vi "CRYPost Processing.vi"(0 "Setup in":T1={"No.VI"=0, "Category"="", "StepName"="", "Seq setup flattened"="", "Comment"="", "Steps config."=[], "Jump config"=[], "Start"=0.0, "Increment"=0.0, "Name"="Pa", "Unit"="Pa", "Y data"=1, "Y prefix"="", "Y dB ref"=1.0, "Y unit"="", "Repeat State Array"=[]} {"Repeat State Array"."Start" format="%#_5g"; "Y dB ref" format="%.1f"; "Y data" items=["dB", "Lin"]; "Start" format="%#_5g"}, 5 "Data in":T4[](array[typedef]) {"Z data" items=["dB", "Lin"]; "X data" items=["dB", "Lin"]; "Y data" items=["dB", "Lin"]; "Z dB ref" format="%.1f"; "Z axis" items=["Log", "Lin"]; "X dB ref" format="%.1f"; "X axis" items=["Log", "Lin"]; "Y axis" items=["Log", "Lin"]; "Y dB ref" format="%.1f"; "Curve"."z" format="%.2f"; "Curve"."y" format="%.2f"; "Curve"."x" format="%.2f"}, 7 "Results in":T5 {"Margin" format="%.2f"}, 9 "Seq Setup in":string, 11 "Step name":string, 12 "Hardware in":string, 13 "Calibration in":string) -> (3 "Types Out":string[](array[string]), 4 "Inserted Names Out":string[](array[string]), 6 "Data out":T3 {"Z data" items=["dB", "Lin"]; "X data" items=["dB", "Lin"]; "Y data" items=["dB", "Lin"]; "Z dB ref" format="%.1f"; "Z axis" items=["Log", "Lin"]; "X dB ref" format="%.1f"; "X axis" items=["Log", "Lin"]; "Y axis" items=["Log", "Lin"]; "Y dB ref" format="%.1f"; "Curve"."z" format="%.2f"; "Curve"."y" format="%.2f"; "Curve"."x" format="%.2f"}, 8 "Result Out":T5 {"Margin" format="%.2f"}, 10 "Wave out":T7 {"Y dB ref" format="%.1f"; "Y axis" items=["Log", "Lin"]; "Y data" items=["dB", "Lin"]; "X data" items=["dB", "Lin"]})   [LabVIEW 2013]
uses:
  Typedef Control/CRYData Cluster.ctl
  Typedef Control/CRYResult Cluster Array.ctl
  Typedef Control/CRYResult Cluster.ctl
  Typedef Control/CRYWaveform Cluster Array.ctl
  Typedef Control/CRYWaveform Cluster.ctl
  Typedef Control/CRYData Cluster Array.ctl
  Typedef Control/CRYStep.ctl
  Task Sequence/CRYProject Run Control Global.vi
  CRYMainGlobal.vi
  SubVI/CRYPost Processing Global.vi
panel:
  in  "output cluster":T2
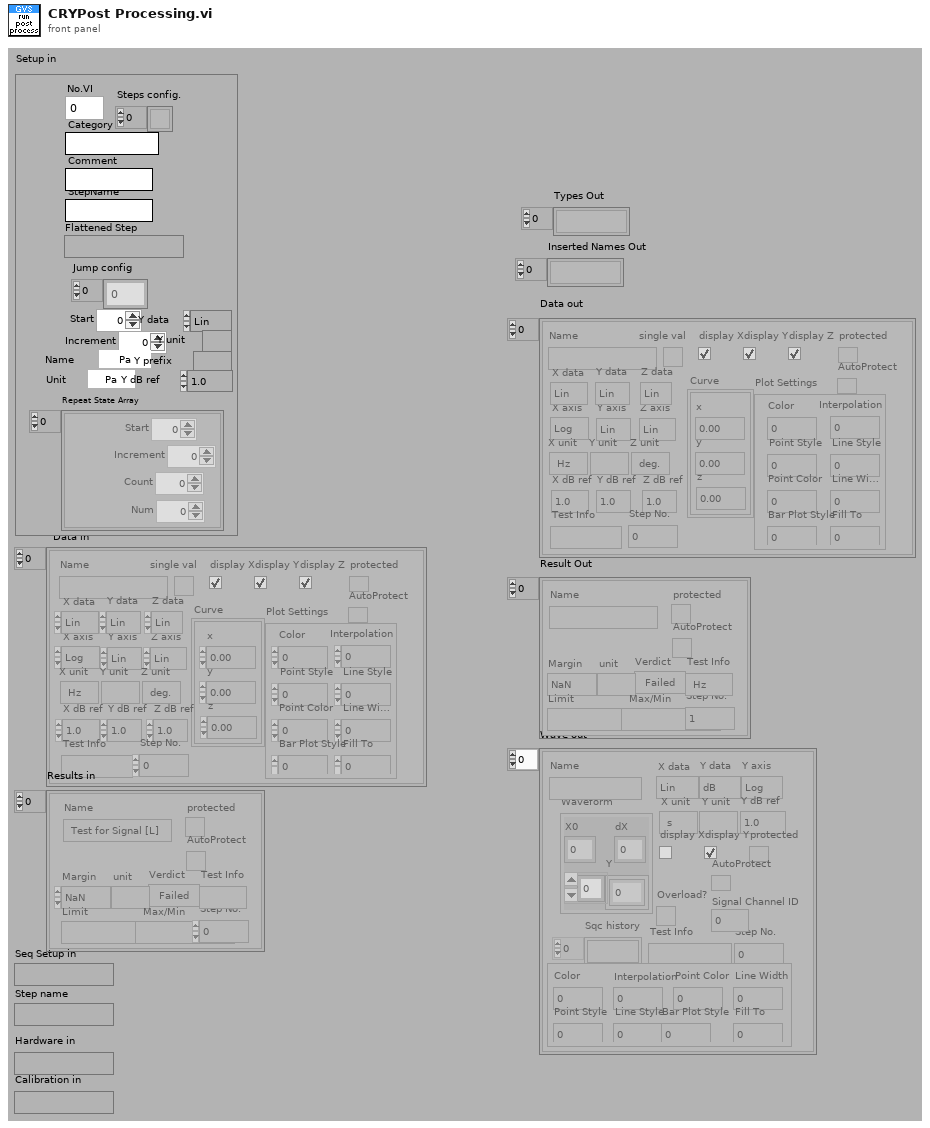
[diagram p1: front panel]
types:
  T1 = typedef "CRYStep.ctl" = cluster{"No.VI":i32, "Category":string, "StepName":string, "Seq setup flattened":string, "Comment":string, "Steps config.":bool[], "Jump config":i32[], "Start":dbl, "Increment":dbl, "Name":string, "Unit":string, "Y data":u16, "Y prefix":string, "Y dB ref":dbl, "Y unit":string, "Repeat State Array":cluster{"Start":dbl, "Increment":dbl, "Count":i32, "Num":i32}[]}
  T2 = cluster{"Res Name":string, "Type out":enum16{"Curves", "Values", "Results", "WFM"}}
  T3 = typedef "CRYData Cluster Array.ctl" = T4[]
  T4 = typedef "CRYData Cluster.ctl" = cluster{"Name":string, "Curve":cluster{"x":dbl, "y":dbl, "z":dbl}[], "X data":u16, "Y data":u16, "Z data":u16, "X axis":u16, "Y axis":u16, "Z axis":u16, "X unit":string, "Y unit":string, "Z unit":string, "X dB ref":dbl, "Y dB ref":dbl, "Z dB ref":dbl, "single val":bool, "protected":bool, "display X":bool, "display Y":bool, "display Z":bool, "Test Info":string, "Step No.":i32, "Plot Settings":cluster{"Color":u32, "Interpolation":u8, "Point Style":u8, "Line Style":u8, "Point Color":u32, "Line Width":u8, "Bar Plot Style":u8, "Fill To":i16}, "AutoProtect":bool}
  T5 = typedef "CRYResult Cluster Array.ctl" = T6[]
  T6 = typedef "CRYResult Cluster.ctl" = cluster{"Name":string, "Margin":dbl, "unit":string, "Verdict":bool, "Limit":string, "Max/Min":string, "protected":bool, "Step No.":i32, "Test Info":string, "AutoProtect":bool}
  T7 = typedef "CRYWaveform Cluster Array.ctl" = T8[]
  T8 = typedef "CRYWaveform Cluster.ctl" = cluster{"Waveform":cluster{"X0":dbl, "dX":dbl, "Y":sgl[]}, "X data":u16, "Y data":u16, "Y axis":u16, "X unit":string, "Y unit":string, "Y dB ref":dbl, "display Y":bool, "display X":bool, "Overload?":bool, "Test Info":string, "Step No.":i32, "Name":string, "protected":bool, "Sqc history":string[], "Signal Channel ID":i32, "Plot Settings":cluster{"Color":u32, "Interpolation":u8, "Point Style":u8, "Line Style":u8, "Point Color":u32, "Line Width":u8, "Bar Plot Style":u8, "Fill To":i16}, "AutoProtect":bool}
  T9 = cluster{"variant":variant, "Overwrite":bool, "Old Name":string, "New Name":string}
  T10 = cluster{"Start":dbl, "Increment":dbl, "Count":i32, "Num":i32}[]
  T11 = typedef "CRYPost Processing Cluster.ctl" = cluster{"Name":string, "Op Type":u16, "Curve A":string, "Curve B":string, "Axis Mode":u16, "Work Mode":u16, "Width":u16, "Weighting win":u16, "Search Mode":u16, "Freq Mode":u16, "New Sampling Rate":dbl, "Use Default Name":bool, "x":bool, "y":bool, "z":bool, "All points":bool, "A_single val axis":u16, "B_single val axis":u16, "Use Default Value":bool, "Result Name":string, "Smoothing Width":i32, "Window":u16, "Para_dB":sgl, "Para_%":sgl, "Exponent":sgl, "Hz":dbl, "Direct Weighting":bool, "Auto Inc":bool, "Inc(deg)":i32, "Total Rotation":i32, "Ref Freq Mode":u16, "Ref Waveform":string, "Sampling Rate":dbl, "Weighting Curve":string, "Ref Freq":dbl, "Curve Group":string[], "Search Items":string[], "Custom unit info":cluster{"use custom":bool, "lin/log":u16, "unit":string, "dB ref":dbl, "common dB":u16}, "Unit":string, "Type A":enum16{"Curves", "Values", "Results", "WFM"}, "Type B":enum16{"Curves", "Values", "Results", "WFM"}, "Unary Operator":u16, "Binary Operator":u16, "Statistical Operator":u16, "Constant ":dbl, "New Resolution":u16, "user equation cluster":T12, "Help":string, "Tab Value":enum32{"Setting", "Help"}, "Zwciker_X-axis":u16, "Zwicker_spectrum":bool, "Freq Sampling Mode":u16, "Freq Sampling Rate":dbl, "Smoothing":bool, "Work in Statics":u16, "Result Data":string[]}
  T12 = typedef "CRYUser Equation Cluster.ctl" = cluster{"Custom unit input array":cluster{"use custom":bool, "lin/log":u16, "unit":string, "dB ref":dbl, "common dB":u16}[], "Custom unit results array ":cluster{"use custom":bool, "lin/log":u16, "unit":string, "dB ref":dbl, "common dB":u16}[], "Desired Result Variables":string[], "Desired Result Names":string[], "Input Curve Names":string[], "Input Curve Variables":string[], "equation":string, "Input axis":u16[], "Results axis":u16[], "# input curves":i32, "# Desired result curves ":i32, "Input Values":string[], "Result Values":string[]}
  T13 = cluster{"Res Name":string, "Type out":enum16{"Curves", "Values", "Results", "WFM"}}[]
  T14 = enum16{"OK", "Yes", "YesNo", "YesNoCancel", "ReplaceAppend"}
  T15 = cluster{"variant":variant, "Overwrite":bool, "Old Name":string, "New Name":string}[]
  T16 = cluster{"use custom":bool, "lin/log":u16, "unit":string, "dB ref":dbl, "common dB":u16}
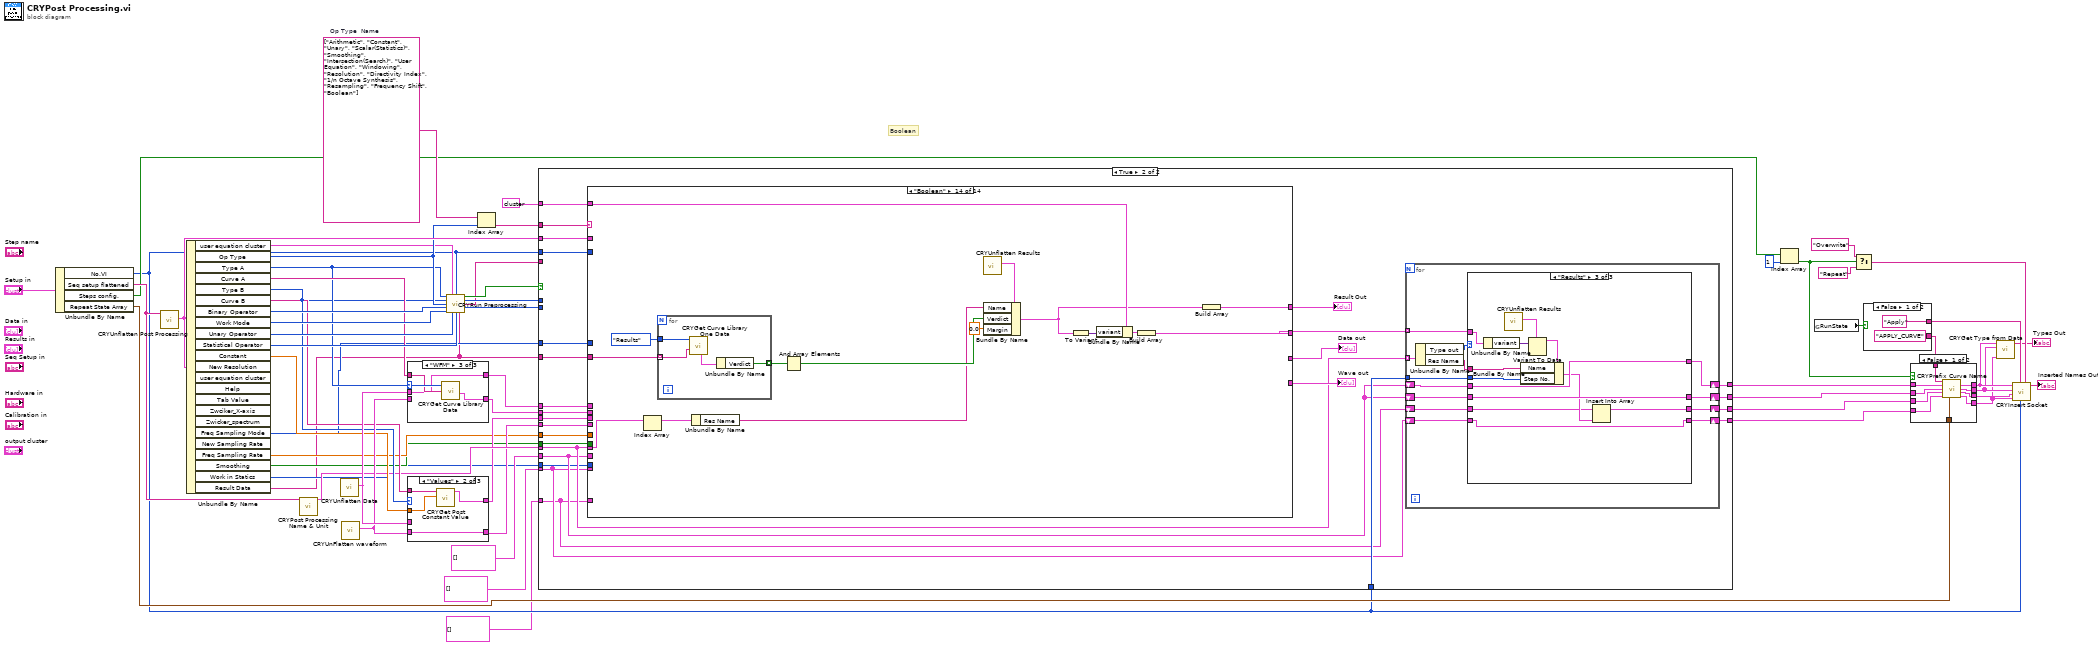
[diagram p0: block diagram]
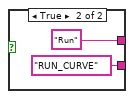
[diagram p2: hidden frame]
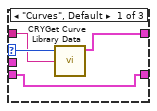
[diagram p4: hidden frame]
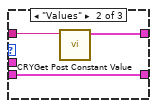
[diagram p5: hidden frame]
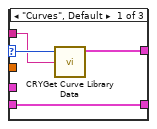
[diagram p6: hidden frame]
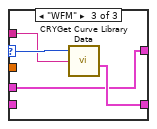
[diagram p7: hidden frame]
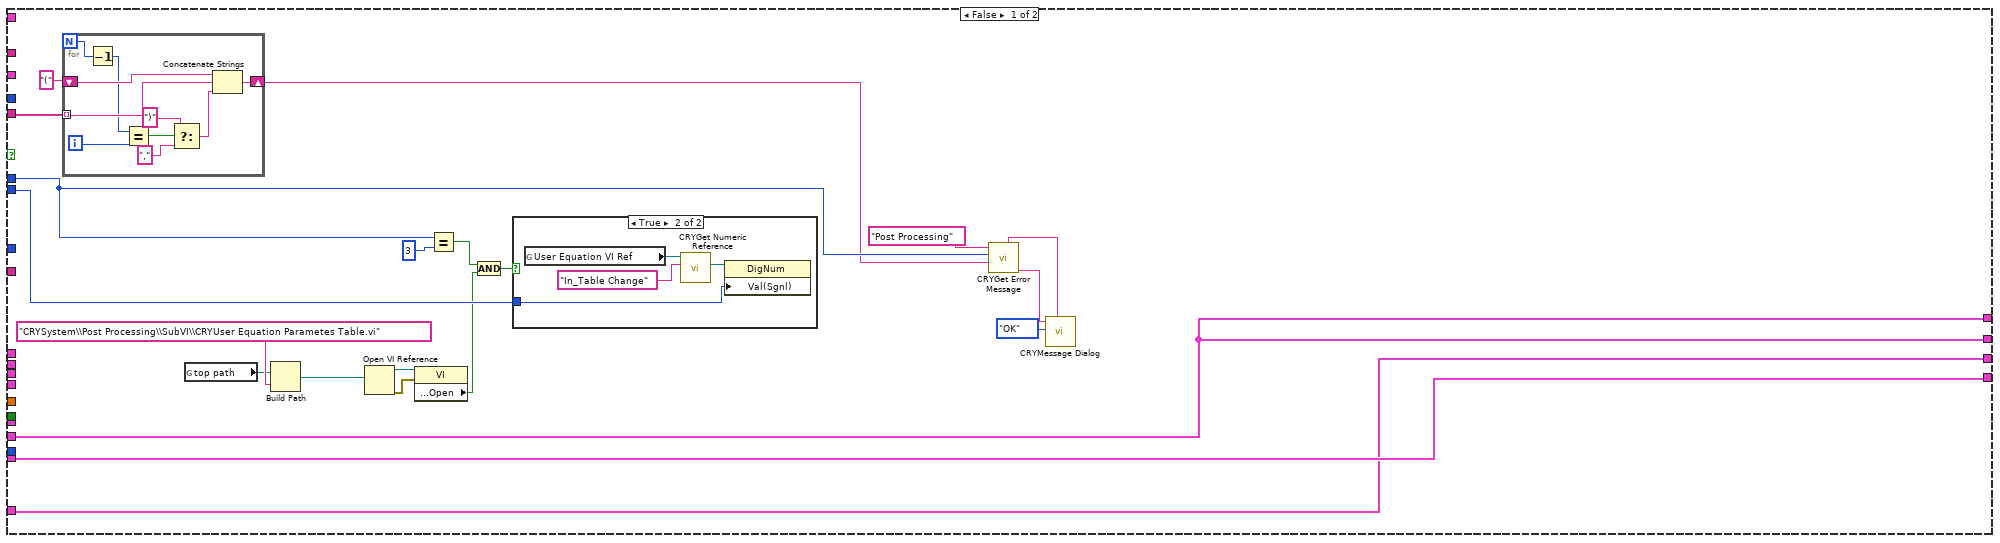
[diagram p8: hidden frame]
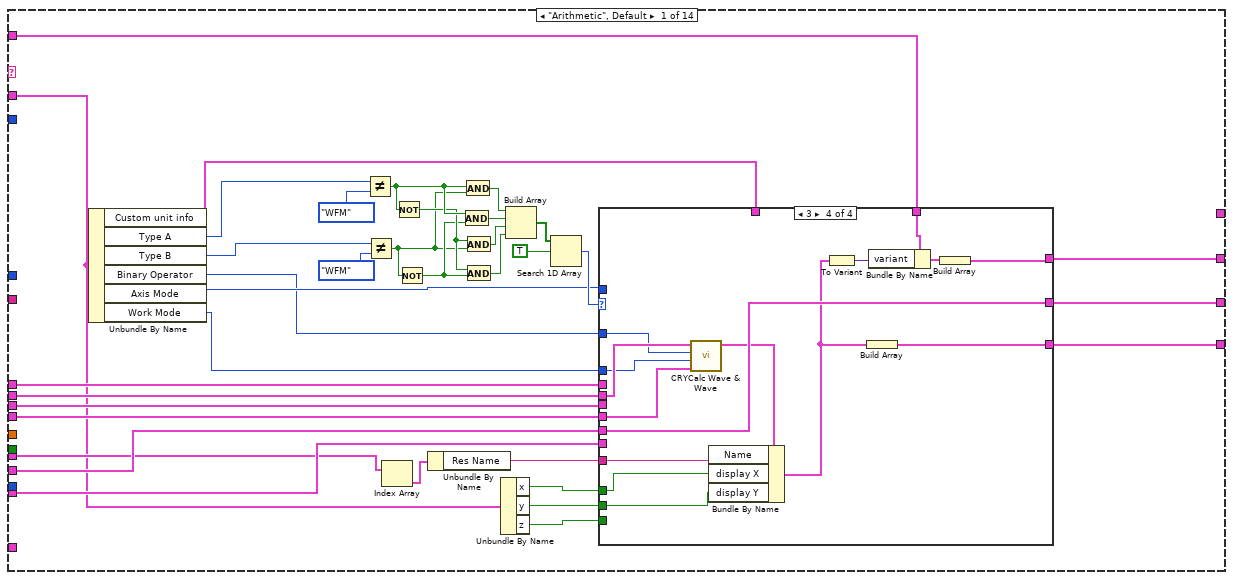
[diagram p10: hidden frame]
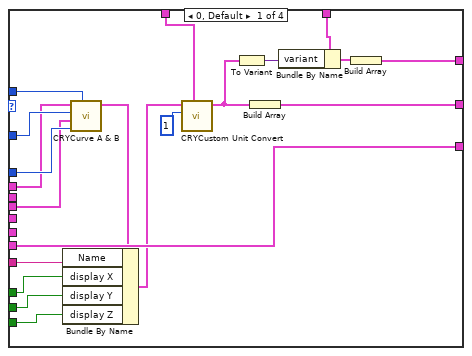
[diagram p11: hidden frame]
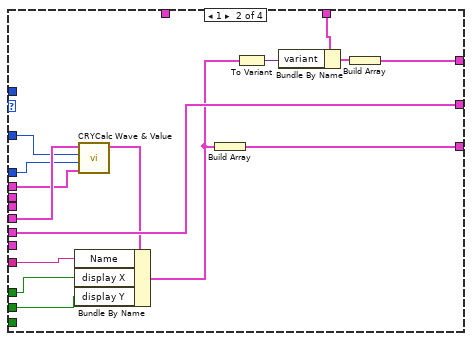
[diagram p12: hidden frame]
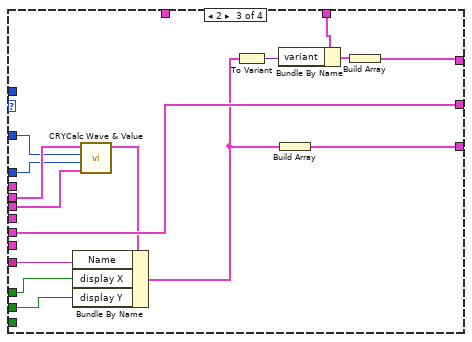
[diagram p13: hidden frame]
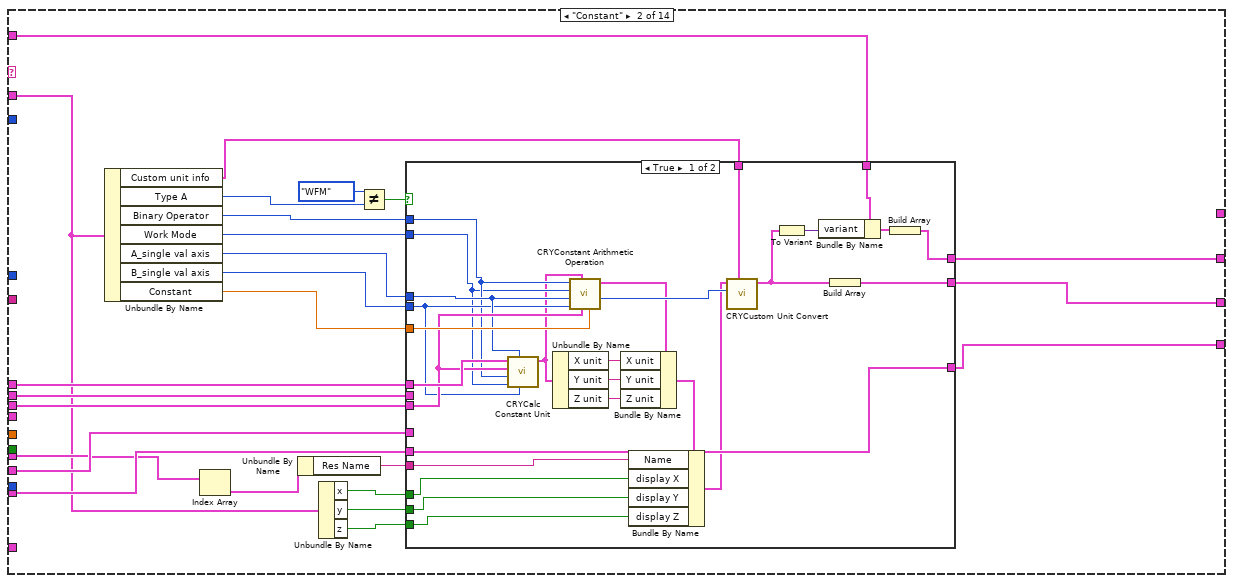
[diagram p14: hidden frame]
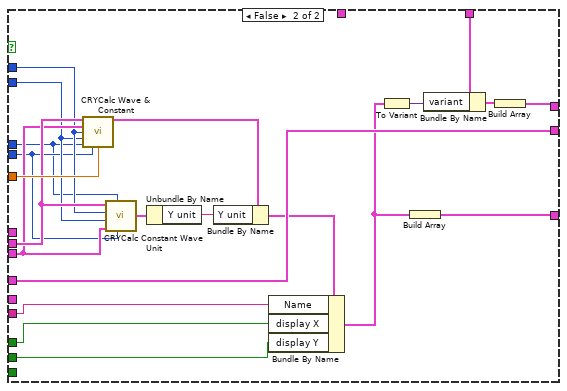
[diagram p15: hidden frame]
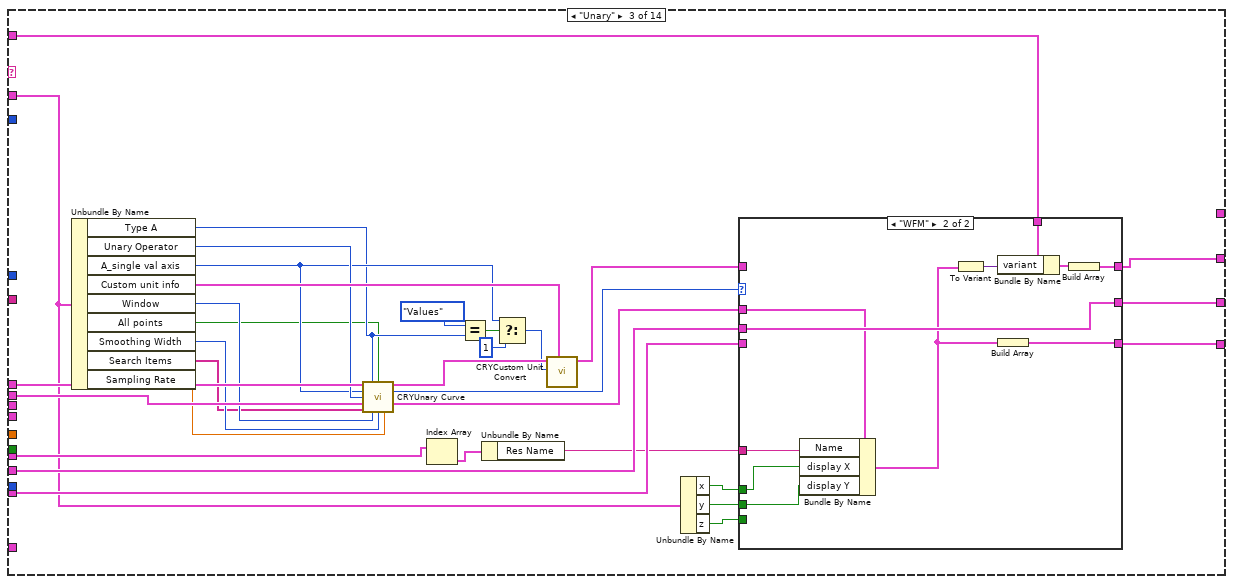
[diagram p16: hidden frame]
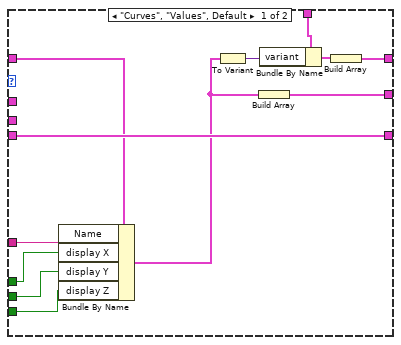
[diagram p17: hidden frame]
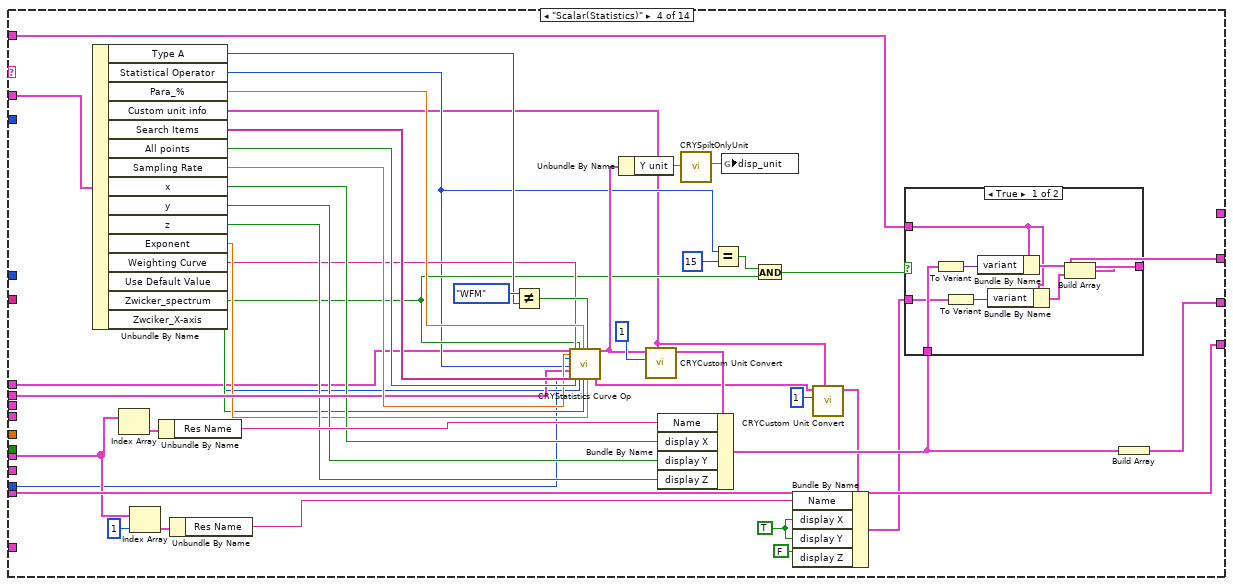
[diagram p18: hidden frame]
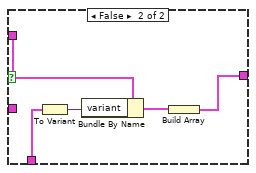
[diagram p19: hidden frame]
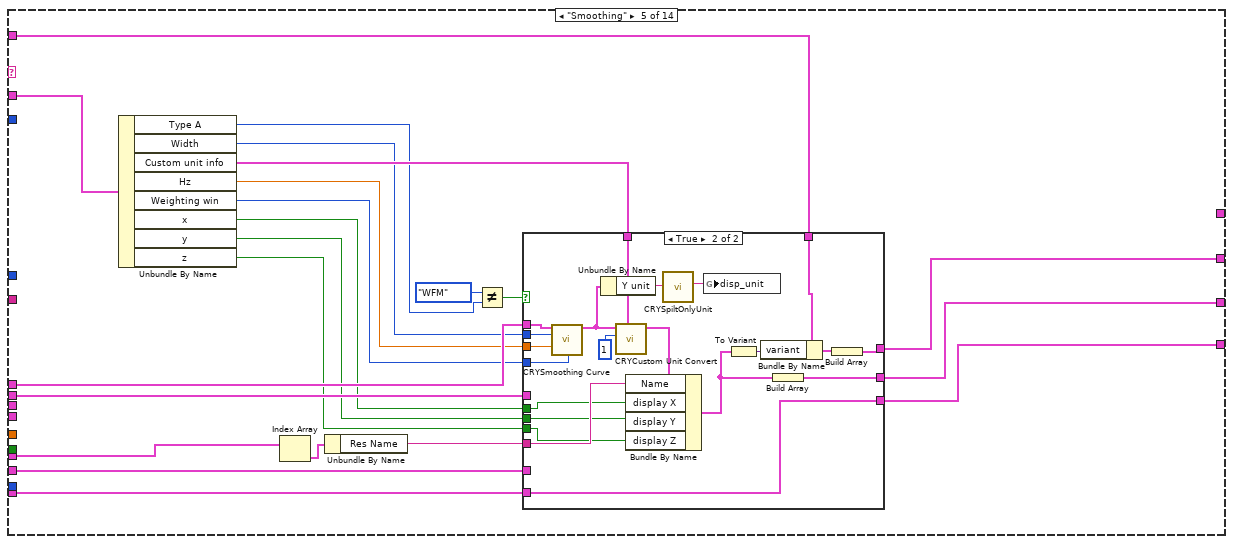
[diagram p20: hidden frame]
diagram:
  w56 = string[] ["Arithmetic", "Constant", "Unary", "Scalar(Statistics)", "Smoothing", "Intersection(Search)", "User Equation", "Windowing", "Resolution", "Directivity Index", "1/n Octave Synthesis", "Resampling", "Frequency Shift", "Boolean"]  # Op Type  Name
  # "Boolean"
  n1 = Unbundle By Name("Setup in") -> ("No.VI"=w9:i32, "Seq setup flattened"=w32:string, "Steps config."=w28:bool[], "Repeat State Array"=w18:T10)
  n2 = call "CRYUnflatten Post Processing.vi"("Unflatten Post Processing"=w32) -> ("Post-Processing"=w50:T11)  [unwired: 10 out]
  n3 = Unbundle By Name(w50) -> ("user equation cluster"=w47:T12, "Op Type"=w48:u16, "Type A"=w38:enum16{"Curves", "Values", "Results", "WFM"}, "Curve A"=w39:string, "Type B"=w36:enum16{"Curves", "Values", "Results", "WFM"}, "Curve B"=w37:string, "Binary Operator"=w55:u16, "Work Mode"=w54:u16, "Unary Operator"=w53:u16, "Statistical Operator"=w52:u16, "Constant"=w35:dbl, "Freq Sampling Mode"=w8:u16, "Freq Sampling Rate"=w7:dbl, "Smoothing"=w6:bool, "Work in Statics"=w5:u16, "Result Data"=w1:string[])  [unwired: 7 out]
  n4 = call "CRYPost Processing Name & Unit.vi"("Step setup"=w32) -> ("Result name and type"=w34:T13)  [unwired: 6 in, 4 out]
  n5 = call "CRYUnflatten Data.vi"() -> ("Datum"=w41:T4)  [unwired: 9 in, 2 out]
  n6 = call "CRYUnFlatten waveform.vi"() -> ("Waveform Cluster"=w40:T8)  [unwired: 9 in, 2 out]
  n7 = case shown="\"WFM\"" w38 {
    selector: w38 -> [w61 _ w68]
    tunnel: w39 -> [w60 w64 w67]
    tunnel: [w59 w63 w65] -> w26
    tunnel: w40 -> [w58 w62 _]
    tunnel: w41 -> [_ _ w65]
    tunnel: [w58 w62 w66] -> w25
    frame "Curves", Default {
      n8 = call "CRYGet Curve Library Data.vi"("Type"=w61, "Data Name"=w60) -> ("Curve"=w59:T4)  [unwired: 4 out]
    }
    frame "Values" {
      n9 = call "CRYGet Post Constant Value.vi"("Data Name"=w64) -> ("Value"=w63:T4)  [unwired: 2 in, 8 out]
    }
    frame "WFM" {
      n10 = call "CRYGet Curve Library Data.vi"("Type"=w68, "Data Name"=w67) -> ("Wave"=w66:T8)  [unwired: 4 out]
    }
  }
  n11 = case shown="\"Values\"" w36 {
    selector: w36 -> [w72 _ w80]
    tunnel: w37 -> [w71 w76 w79]
    tunnel: w35 -> [_ w75 _]
    tunnel: w41 -> [_ _ w77]
    tunnel: w40 -> [w69 w73 _]
    tunnel: [w70 w74 w77] -> w24
    tunnel: [w69 w73 w78] -> w23
    frame "Curves", Default {
      n12 = call "CRYGet Curve Library Data.vi"("Type"=w72, "Data Name"=w71) -> ("Curve"=w70:T4)  [unwired: 4 out]
    }
    frame "Values" {
      n13 = call "CRYGet Post Constant Value.vi"("Constant"=w75, "Data Name"=w76) -> ("Value"=w74:T4)  [unwired: 1 in, 8 out]
    }
    frame "WFM" {
      n14 = call "CRYGet Curve Library Data.vi"("Type"=w80, "Data Name"=w79) -> ("Wave"=w78:T8)  [unwired: 4 out]
    }
  }
  n15 = call "CRYRun Preprocessing.vi"("Type A"=w38, "user equation cluster"=w47, "No.VI"=w9, "Type B"=w36, "Type"=w48, "Binary Operator"=w55, "Work in"=w54, "Unary Operator"=w53, "Statistical Operator"=w52, "Result Data"=w1) -> ("Run Flag"=w51:bool, "Message Mode"=w49:u16, "Invalid Variable"=w46:string[], "index of Invalid"=w45:i32)  [unwired: 2 out]
  n16 = Index Array(array=w56, index=w48) -> (element=w57:string)
  n17 = case shown="True" w51 {
    tunnel: w57 -> [_ w141]
    tunnel: w50 -> [_ w140]
    tunnel: w26 -> [_ w139]
    tunnel: w25 -> [_ w138]
    tunnel: w24 -> [_ w137]
    tunnel: w23 -> [_ w136]
    tunnel: w49 -> [w96 _]
    tunnel: w46 -> [w100 _]
    tunnel: w45 -> [w98 _]
    tunnel: T4[] [] ("appended array") -> [w82 w126]
    tunnel: T8[] [] ("appended array") -> [w83 w125]
    tunnel: T9 {"variant"=variant, "Overwrite"=FALSE, "Old Name"="", "New Name"=""} ("Data") -> [_ w133]
    tunnel: w34 -> [_ w131]
    tunnel: [w82 w130] -> w22
    tunnel: [w82 w129] -> w21
    tunnel: [w83 w128] -> w20
    tunnel: w9 -> [_ w127]
    tunnel: w9 -> [_ w124]
    tunnel: w8 -> [_ w123]
    tunnel: w7 -> [_ w122]
    tunnel: w6 -> [_ w121]
    tunnel: w5 -> [_ w120]
    tunnel: T6[] [] ("appended array") -> [w81 w116]
    tunnel: [w81 w119] -> w3
    tunnel: w1 -> [_ w118]
    frame False {
      n18 = for {
        N -> [w112]
        tunnel: w100 -> [w115] mode=indexing
        shift-right: [w114] -> w92
        shift-left: "(" ("string") -> [w113]
        i -> [w111]
        n19 = Decrement(x=w112) -> (x-1=w110:i32)
        n20 = Equal?(x=w110, y=w111) -> (x = y?=w109:bool)
        n21 = Select(t=")", s=w109, f="," ("string")) -> (s? t:f=w106:string)
        n22 = Concatenate Strings(w113, w115, w106) -> (w114:string)
      }
      n23 = global read "CRYMainGlobal.vi" "top path"() -> (w89:path)
      n24 = Build Path(base path=w89, name or relative path="CRYSystem\\Post Processing\\SubVI\\CRYUser Equation Parametes Table.vi" ("StepName")) -> (appended path=w91:path)
      n25 = Open VI Reference(vi path=w91) -> (vi reference=w85:refnum<vi>, error out=w84:errorcluster)  [unwired: 1 in, 4 out]
      n26 = property class="VI"(reference=w85, error in=w84) -> ("Front Panel.Open"=w88:bool)  [unwired: 2 out]
      n27 = Equal?(x=w96, y=u16 3) -> (x = y?=w87:bool)
      n28 = And(x=w87, y=w88) -> (x .and. y?=w86:bool)
      n29 = case shown="True" w86 {
        tunnel: w98 -> [_ w102]
        frame False {
        }
        frame True {
          n30 = global read "CRYPost Processing Global.vi" "User Equation VI Ref"() -> (w105:refnum<vi>)
          n31 = call "CRYGet Numeric Reference.vi"("Label Name"="In_Table Change", "VI Refnum"=w105) -> ("Numeric Ref Out"=w103:refnum<vi>)  [unwired: 7 in, 2 out]
          n32 = property class="DigNum"(reference=w103, "Val(Sgnl)"=w102) -> ()  [unwired: 1 in, 2 out]
        }
      }
      n33 = call "CRYGet Error Message.vi"("String In"=w92, "Error No"=w96, "Kind"="Post Processing") -> ("Message Sub 3"=w95:string, "Window Title"=w94:string)  [unwired: 3 in, 4 out]
      n34 = call "CRYMessage Dialog.vi"("Window Title"=w94, "YesNoCancel"=T14."OK", "Message Content"=w95) -> ()  [unwired: 7 in, 2 out]
    }
    frame True {
      n35 = case shown="\"Boolean\"" w141 {
        tunnel: w140 -> [w145 w246 w318 w415 w450 w497 w563 w620 w751 w777 w799 w818 w873 _]
        tunnel: w139 -> [w159 w262 w343 w382 w449 w530 _ w617 w728 w755 w797 _ _ _]
        tunnel: w138 -> [w158 w261 w346 w408 w440 w511 _ w616 _ _ _ w811 w853 _]
        tunnel: w137 -> [w157 w260 _ _ _ w528 _ _ _ _ _ _ _ _]
        tunnel: w136 -> [w156 _ _ _ _ w512 _ _ _ _ _ _ _ _]
        tunnel: [w151 w256 w328 w404 w442 w508 w573 w611 w745 w774 w794 w817 w872 _] -> w135
        tunnel: [w155 w255 w326 w403 w439 w507 w567 w610 w744 w773 w793 w801 w850 _] -> w134
        tunnel: w126 -> [w152 w252 w325 _ w437 _ _ w613 _ _ _ w817 w868 _]
        tunnel: w125 -> [w153 w253 w327 w403 w438 w507 w567 w614 w744 w773 w793 w809 w867 _]
        tunnel: w133 -> [w150 w251 w330 w402 w436 w503 w572 w609 w741 w770 w790 w816 w871 w998]
        tunnel: [w149 w250 w329 w400 w435 w504 w571 w608 w740 w769 w789 w815 w870 w997] -> w132
        tunnel: w131 -> [w148 w249 w324 w377 w434 w502 _ w607 w739 w767 w787 w813 w857 w987]
        tunnel: w124 -> [_ _ _ _ _ _ w562 _ _ _ _ _ _ _]
        tunnel: w123 -> [_ _ _ _ _ _ _ _ _ _ _ _ w848 _]
        tunnel: w122 -> [_ _ _ _ _ _ _ _ _ _ _ _ w847 _]
        tunnel: w121 -> [_ _ _ _ _ _ _ _ w727 _ _ _ _ _]
        tunnel: w120 -> [_ _ _ w370 _ _ _ _ _ _ _ _ _ _]
        tunnel: w118 -> [_ _ _ _ _ _ _ _ _ _ _ _ _ w990]
        tunnel: [_ _ _ _ _ _ _ _ _ _ _ _ _ w992] -> w117
        tunnel: w116 -> [_ _ _ _ _ _ _ _ _ _ _ _ _ _]
        frame "Arithmetic", Default {
          n36 = Unbundle By Name(w145) -> ("Custom unit info"=w154:T16, "Type A"=w165:enum16{"Curves", "Values", "Results", "WFM"}, "Type B"=w164:enum16{"Curves", "Values", "Results", "WFM"}, "Binary Operator"=w161:u16, "Axis Mode"=w162:u16, "Work Mode"=w160:u16)
          n37 = Not Equal?(x=w165, y=enum16{"Curves", "Values", "Results", "WFM"}."WFM" ("Type A")) -> (x != y?=w174:bool)
          n38 = Not Equal?(x=w164, y=enum16{"Curves", "Values", "Results", "WFM"}."WFM" ("Type A")) -> (x != y?=w171:bool)
          n39 = Index Array(array=w148) -> (element=w147:T2)  [unwired: 1 in]
          n40 = Not(x=w174) -> (.not. x?=w173:bool)
          n41 = Not(x=w171) -> (.not. x?=w172:bool)
          n42 = Unbundle By Name(w147) -> ("Res Name"=w146:string)
          n43 = And(x=w174, y=w172) -> (x .and. y?=w170:bool)
          n44 = And(x=w174, y=w171) -> (x .and. y?=w177:bool)
          n45 = And(x=w173, y=w171) -> (x .and. y?=w169:bool)
          n46 = And(x=w173, y=w172) -> (x .and. y?=w168:bool)
          n47 = Unbundle By Name(w145) -> ("x"=w144:bool, "y"=w143:bool, "z"=w142:bool)
          n48 = Build Array(w177, w170, w169, w168) -> (w176:bool[])
          n49 = Search 1D Array(1D array=w176, element=TRUE) -> (index of element=w163:i32)  [unwired: 1 out]
          n50 = case shown="3" w163 {
            tunnel: w159 -> [w194 w211 _ _]
            tunnel: w158 -> [_ _ w227 w242]
            tunnel: w157 -> [w193 _ w226 _]
            tunnel: w156 -> [_ w212 _ w241]
            tunnel: w161 -> [w196 w210 w225 w240]
            tunnel: w162 -> [w197 _ _ _]
            tunnel: w160 -> [w195 w209 w224 w239]
            tunnel: w154 -> [w192 _ _ _]
            tunnel: [w189 w208 w223 w238] -> w155
            tunnel: [w190 w207 w222 w237] -> w151
            tunnel: w153 -> [w189 _ _ _]
            tunnel: w152 -> [_ w207 w222 w237]
            tunnel: w150 -> [w188 w204 w219 w234]
            tunnel: [w184 w203 w218 w233] -> w149
            tunnel: w146 -> [w182 w201 w216 w231]
            tunnel: w144 -> [w180 w199 w214 w229]
            tunnel: w143 -> [w179 w198 w213 w228]
            tunnel: w142 -> [w178 _ _ _]
            frame 0, Default {
              n51 = call "CRYCurve A & B.vi"("X-axis Combination"=w197, "Work in"=w195, "Curve B"=w193, "Operator"=w196, "Curve A"=w194) -> ("Result"=w183:T4)  [unwired: 6 out]
              n52 = Bundle By Name(cluster=w183, "Name"=w182, "display X"=w180, "display Y"=w179, "display Z"=w178) -> (w181:T4)
              n53 = call "CRYCustom Unit Convert.vi"("Custom unit info"=w192, "Axis Mode"=u16 1, "Data in"=w181) -> ("Data out"=w187:T4)  [unwired: 8 out]
              n54 = To Variant(anything=w187) -> (Variant=w186:variant)
              n55 = Build Array(w187) -> (w190:T4[])
              n56 = Bundle By Name(cluster=w188, "variant"=w186) -> (w185:T9)
              n57 = Build Array(w185) -> (w184:T15)
            }
            frame 1 {
              n58 = call "CRYCalc Wave & Value.vi"("Value in"=w211, "Work in"=w209, "Operator"=w210, "Wave in"=w212) -> ("Wave out"=w202:T8)  [unwired: 7 out]
              n59 = Bundle By Name(cluster=w202, "Name"=w201, "display X"=w199, "display Y"=w198) -> (w200:T8)
              n60 = Build Array(w200) -> (w208:T8[])
              n61 = To Variant(anything=w200) -> (Variant=w206:variant)
              n62 = Bundle By Name(cluster=w204, "variant"=w206) -> (w205:T9)
              n63 = Build Array(w205) -> (w203:T15)
            }
            frame 2 {
              n64 = call "CRYCalc Wave & Value.vi"("Value in"=w226, "Work in"=w224, "Operator"=w225, "Wave in"=w227) -> ("Wave out"=w217:T8)  [unwired: 7 out]
              n65 = Bundle By Name(cluster=w217, "Name"=w216, "display X"=w214, "display Y"=w213) -> (w215:T8)
              n66 = To Variant(anything=w215) -> (Variant=w221:variant)
              n67 = Bundle By Name(cluster=w219, "variant"=w221) -> (w220:T9)
              n68 = Build Array(w215) -> (w223:T8[])
              n69 = Build Array(w220) -> (w218:T15)
            }
            frame 3 {
              n70 = call "CRYCalc Wave & Wave.vi"("Wave in_2"=w241, "Work in"=w239, "Operator"=w240, "Wave in_1"=w242) -> ("Wave out"=w232:T8)  [unwired: 7 out]
              n71 = Bundle By Name(cluster=w232, "Name"=w231, "display X"=w229, "display Y"=w228) -> (w230:T8)
              n72 = To Variant(anything=w230) -> (Variant=w236:variant)
              n73 = Build Array(w230) -> (w238:T8[])
              n74 = Bundle By Name(cluster=w234, "variant"=w236) -> (w235:T9)
              n75 = Build Array(w235) -> (w233:T15)
            }
          }
        }
        frame "Constant" {
          n76 = Unbundle By Name(w246) -> ("Custom unit info"=w254:T16, "Type A"=w266:enum16{"Curves", "Values", "Results", "WFM"}, "Binary Operator"=w264:u16, "Work Mode"=w263:u16, "A_single val axis"=w258:u16, "B_single val axis"=w257:u16, "Constant"=w259:dbl)
          n77 = Index Array(array=w249) -> (element=w248:T2)  [unwired: 1 in]
          n78 = Unbundle By Name(w248) -> ("Res Name"=w247:string)
          n79 = Unbundle By Name(w246) -> ("x"=w245:bool, "y"=w244:bool, "z"=w243:bool)
          n80 = Not Equal?(x=enum16{"Curves", "Values", "Results", "WFM"}."WFM" ("Type A"), y=w266) -> (x != y?=w265:bool)
          n81 = case shown="True" w265 {
            tunnel: w262 -> [w291 _]
            tunnel: w261 -> [_ w303]
            tunnel: w260 -> [w290 w302]
            tunnel: w264 -> [w287 w301]
            tunnel: w263 -> [w286 w300]
            tunnel: w258 -> [w289 w298]
            tunnel: w257 -> [w288 w299]
            tunnel: w259 -> [w292 w314]
            tunnel: w254 -> [w293 _]
            tunnel: [w281 w312] -> w256
            tunnel: [w280 w313] -> w255
            tunnel: w253 -> [w280 _]
            tunnel: w252 -> [_ w312]
            tunnel: w251 -> [w277 w309]
            tunnel: [w275 w308] -> w250
            tunnel: w247 -> [w273 w307]
            tunnel: w245 -> [w271 w306]
            tunnel: w244 -> [w270 w305]
            tunnel: w243 -> [w269 _]
            frame True {
              n82 = call "CRYCalc Constant Unit.vi"("B_axis mode"=w288, "A_axis mode"=w289, "Work in"=w286, "Operator"=w287, "B data for units"=w290, "A data for units"=w291) -> ("Result out"=w268:T4)  [unwired: 5 in]
              n83 = Unbundle By Name(w268) -> ("X unit"=w284:string, "Y unit"=w283:string, "Z unit"=w282:string)
              n84 = call "CRYConstant Arithmetic Operation.vi"("Constant"=w292, "B data for units"=w290, "A data for units"=w268, "B_axis mode"=w288, "A_axis mode"=w289, "Work in"=w286, "Operator"=w287) -> ("Result out"=w285:T4)  [unwired: 4 in]
              n85 = Bundle By Name(cluster=w285, "X unit"=w284, "Y unit"=w283, "Z unit"=w282) -> (w274:T4)
              n86 = Bundle By Name(cluster=w274, "Name"=w273, "display X"=w271, "display Y"=w270, "display Z"=w269) -> (w272:T4)
              n87 = call "CRYCustom Unit Convert.vi"("Custom unit info"=w293, "Axis Mode"=w289, "Data in"=w272) -> ("Data out"=w276:T4)  [unwired: 8 out]
              n88 = To Variant(anything=w276) -> (Variant=w279:variant)
              n89 = Bundle By Name(cluster=w277, "variant"=w279) -> (w278:T9)
              n90 = Build Array(w276) -> (w281:T4[])
              n91 = Build Array(w278) -> (w275:T15)
            }
            frame False {
              n92 = call "CRYCalc Wave & Constant.vi"("Wave in"=w303, "Value in"=w302, "Operator"=w301, "Work in"=w300, "A_axis mode"=w298, "B_axis mode"=w299, "Constant"=w314) -> ("Wave out"=w296:T8)  [unwired: 8 out]
              n93 = call "CRYCalc Constant Wave Unit.vi"("B_axis mode"=w299, "A_axis mode"=w298, "Value in"=w302, "Work in"=w300, "Operator"=w301, "Wave in"=w303) -> ("Wave out"=w297:T8)  [unwired: 5 in]
              n94 = Unbundle By Name(w297) -> ("Y unit"=w295:string)
              n95 = Bundle By Name(cluster=w296, "Y unit"=w295) -> (w294:T8)
              n96 = Bundle By Name(cluster=w294, "Name"=w307, "display X"=w306, "display Y"=w305) -> (w304:T8)
              n97 = To Variant(anything=w304) -> (Variant=w311:variant)
              n98 = Build Array(w304) -> (w313:T8[])
              n99 = Bundle By Name(cluster=w309, "variant"=w311) -> (w310:T9)
              n100 = Build Array(w310) -> (w308:T15)
            }
          }
        }
        frame "Unary" {
          n101 = Unbundle By Name(w318) -> ("Type A"=w334:enum16{"Curves", "Values", "Results", "WFM"}, "Unary Operator"=w342:u16, "A_single val axis"=w337:u16, "Custom unit info"=w345:T16, "Window"=w341:u16, "All points"=w320:bool, "Smoothing Width"=w340:i32, "Search Items"=w321:string[], "Sampling Rate"=w319:dbl)
          n102 = call "CRYUnary Curve.vi"("Operand A"=w343, "Type A"=w334, "All points"=w320, "A _axis mode"=w337, "Unary Operator"=w342, "Wave in"=w346, "Search Items"=w321, "Win Mode"=w341, "Smoothing Width"=w340, "Sampling Rate"=w319) -> ("Result"=w344:T4, "Type out"=w333:enum16{"Curves", "Values", "Results", "WFM"}, "Wave out"=w331:T8)  [unwired: 3 out]
          n103 = Index Array(array=w324) -> (element=w323:T2)  [unwired: 1 in]
          n104 = Equal?(x=enum16{"Curves", "Values", "Results", "WFM"}."Values", y=w334) -> (x = y?=w338:bool)
          n105 = Unbundle By Name(w323) -> ("Res Name"=w322:string)
          n106 = Select(t=w337, s=w338, f=u16 1) -> (s? t:f=w335:u16)
          n107 = call "CRYCustom Unit Convert.vi"("Custom unit info"=w345, "Axis Mode"=w335, "Data in"=w344) -> ("Data out"=w332:T4)  [unwired: 8 out]
          n108 = Unbundle By Name(w318) -> ("x"=w317:bool, "y"=w316:bool, "z"=w315:bool)
          n109 = case shown="\"WFM\"" w333 {
            tunnel: w332 -> [w352 _]
            tunnel: w331 -> [_ w363]
            tunnel: w330 -> [w356 w367]
            tunnel: [w355 w366] -> w329
            tunnel: [w354 w364] -> w328
            tunnel: w327 -> [w353 _]
            tunnel: [w353 w365] -> w326
            tunnel: w325 -> [_ w364]
            tunnel: w322 -> [w351 w362]
            tunnel: w317 -> [w349 w360]
            tunnel: w316 -> [w348 w359]
            tunnel: w315 -> [w347 _]
            frame "Curves", "Values", Default {
              n110 = Bundle By Name(cluster=w352, "Name"=w351, "display X"=w349, "display Y"=w348, "display Z"=w347) -> (w350:T4)
              n111 = To Variant(anything=w350) -> (Variant=w358:variant)
              n112 = Build Array(w350) -> (w354:T4[])
              n113 = Bundle By Name(cluster=w356, "variant"=w358) -> (w357:T9)
              n114 = Build Array(w357) -> (w355:T15)
            }
            frame "WFM" {
              n115 = Bundle By Name(cluster=w363, "Name"=w362, "display X"=w360, "display Y"=w359) -> (w361:T8)
              n116 = To Variant(anything=w361) -> (Variant=w369:variant)
              n117 = Bundle By Name(cluster=w367, "variant"=w369) -> (w368:T9)
              n118 = Build Array(w361) -> (w365:T8[])
              n119 = Build Array(w368) -> (w366:T15)
            }
          }
        }
        frame "Scalar(Statistics)" {
          w374 = TRUE ("display Y")
          n120 = Unbundle By Name(w415) -> ("Type A"=w410:enum16{"Curves", "Values", "Results", "WFM"}, "Statistical Operator"=w386:u16, "Para_%"=w413:sgl, "Custom unit info"=w379:T16, "Search Items"=w414:string[], "All points"=w412:bool, "Sampling Rate"=w409:dbl, "x"=w397:bool, "y"=w396:bool, "z"=w395:bool, "Exponent"=w391:sgl, "Weighting Curve"=w390:string, "Use Default Value"=w389:bool, "Zwicker_spectrum"=w387:bool, "Zwciker_X-axis"=w388:u16)
          n121 = Index Array(array=w377) -> (element=w399:T2)  [unwired: 1 in]
          n122 = Index Array(array=w377, index=1) -> (element=w378:T2)
          n123 = Unbundle By Name(w399) -> ("Res Name"=w398:string)
          n124 = Unbundle By Name(w378) -> ("Res Name"=w375:string)
          n125 = Not Equal?(x=enum16{"Curves", "Values", "Results", "WFM"}."WFM" ("Type In"), y=w410) -> (x != y?=w407:bool)
          n126 = call "CRYStatistics Curve Op.vi"("Data in"=w382, "Sampling Rate"=w409, "work in statics"=w370, "Statistical Operator"=w386, "Wave"=w408, "Search range"=w414, "weight curve"=w390, "All points"=w412, "Zwicker_spectrum"=w387, "Zwicker_X-axis"=w388, "Para_Resonance(%)"=w413, "Use Default Value"=w389, "Curve/WFM ?"=w407, "Exponent"=w391) -> ("Ranged data out(Curve)"=w380:T4, "Ranged data out(Value)"=w393:T4)  [unwired: 8 in, 4 out]
          n127 = Unbundle By Name(w393) -> ("Y unit"=w392:string)
          n128 = call "CRYCustom Unit Convert.vi"("Custom unit info"=w379, "Axis Mode"=u16 1, "Data in"=w393) -> ("Data out"=w405:T4)  [unwired: 8 out]
          n129 = Bundle By Name(cluster=w405, "Name"=w398, "display X"=w397, "display Y"=w396, "display Z"=w395) -> (w401:T4)
          n130 = call "CRYSpiltOnlyUnit.vi"("In Unit String"=w392) -> ("Out Unit String"=w394:string)  [unwired: 10 in]
          n131 = Equal?(x=w386, y=u16 15) -> (x = y?=w384:bool)
          n132 = global write "CRYPost Processing Global.vi" "disp_unit"(w394) -> ()
          n133 = And(x=w384, y=w387) -> (x .and. y?=w383:bool)
          n134 = call "CRYCustom Unit Convert.vi"("Custom unit info"=w379, "Axis Mode"=u16 1, "Data in"=w380) -> ("Data out"=w373:T4)  [unwired: 8 out]
          n135 = Bundle By Name(cluster=w373, "Name"=w375, "display X"=w374, "display Y"=w374, "display Z"=FALSE) -> (w372:T4)
          n136 = case shown="True" w383 {
            tunnel: w402 -> [w416 w426]
            tunnel: w401 -> [w421 w425]
            tunnel: [w420 w424] -> w400
            tunnel: w372 -> [w418 _]
            frame True {
              n137 = To Variant(anything=w421) -> (Variant=w423:variant)
              n138 = To Variant(anything=w418) -> (Variant=w419:variant)
              n139 = Bundle By Name(cluster=w416, "variant"=w423) -> (w422:T9)
              n140 = Bundle By Name(cluster=w416, "variant"=w419) -> (w417:T9)
              n141 = Build Array(w422, w417) -> (w420:T15)
            }
            frame False {
              n142 = To Variant(anything=w425) -> (Variant=w428:variant)
              n143 = Bundle By Name(cluster=w426, "variant"=w428) -> (w427:T9)
              n144 = Build Array(w427) -> (w424:T15)
            }
          }
          n145 = Build Array(w401) -> (w404:T4[])
        }
        frame "Smoothing" {
          n146 = Unbundle By Name(w450) -> ("Type A"=w444:enum16{"Curves", "Values", "Results", "WFM"}, "Width"=w446:u16, "Custom unit info"=w448:T16, "Hz"=w447:dbl, "Weighting win"=w443:u16, "x"=w431:bool, "y"=w430:bool, "z"=w429:bool)
          n147 = Index Array(array=w434) -> (element=w433:T2)  [unwired: 1 in]
          n148 = Unbundle By Name(w433) -> ("Res Name"=w432:string)
          n149 = Not Equal?(x=enum16{"Curves", "Values", "Results", "WFM"}."WFM" ("Type In"), y=w444) -> (x != y?=w441:bool)
          n150 = case shown="True" w441 {
            tunnel: w449 -> [_ w487]
            tunnel: w448 -> [_ w486]
            tunnel: w447 -> [w464 w485]
            tunnel: w446 -> [_ w484]
            tunnel: w443 -> [w465 w483]
            tunnel: [w462 w481] -> w442
            tunnel: w440 -> [w466 _]
            tunnel: [w463 w480] -> w439
            tunnel: w438 -> [_ w480]
            tunnel: w437 -> [w462 _]
            tunnel: w436 -> [w459 w477]
            tunnel: [w458 w476] -> w435
            tunnel: w432 -> [w457 w474]
            tunnel: w431 -> [w455 w472]
            tunnel: w430 -> [w454 w471]
            tunnel: w429 -> [_ w470]
            frame False {
              n151 = call "CRYSmoothing Waveform.vi"("Weight Mode"=w465, "Width (s)"=w464, "Wave In"=w466) -> ("Wave out"=w451:T8)  [unwired: 8 in]
              n152 = Bundle By Name(cluster=w451, "display X"=w455, "display Y"=w454, "Name"=w457) -> (w456:T8)
              n153 = Unbundle By Name(w451) -> ("Y unit"=w452:string)
              n154 = call "CRYSpiltOnlyUnit.vi"("In Unit String"=w452) -> ("Out Unit String"=w453:string)  [unwired: 10 in]
              n155 = To Variant(anything=w456) -> (Variant=w461:variant)
              n156 = global write "CRYPost Processing Global.vi" "disp_unit"(w453) -> ()
              n157 = Bundle By Name(cluster=w459, "variant"=w461) -> (w460:T9)
              n158 = Build Array(w456) -> (w463:T8[])
              n159 = Build Array(w460) -> (w458:T15)
            }
            frame True {
              n160 = call "CRYSmoothing Curve.vi"("Data in"=w487, "Octav Mode"=w484, "Octave steps"=w485, "Weight Mode"=w483) -> ("Resulting data out"=w467:T4)  [unwired: 2 in, 9 out]
              n161 = Unbundle By Name(w467) -> ("Y unit"=w468:string)
              n162 = call "CRYCustom Unit Convert.vi"("Custom unit info"=w486, "Axis Mode"=u16 1, "Data in"=w467) -> ("Data out"=w475:T4)  [unwired: 8 out]
              n163 = Bundle By Name(cluster=w475, "Name"=w474, "display X"=w472, "display Y"=w471, "display Z"=w470) -> (w473:T4)
              n164 = call "CRYSpiltOnlyUnit.vi"("In Unit String"=w468) -> ("Out Unit String"=w469:string)  [unwired: 10 in]
              n165 = global write "CRYPost Processing Global.vi" "disp_unit"(w469) -> ()
              n166 = To Variant(anything=w473) -> (Variant=w478:variant)
              n167 = Bundle By Name(cluster=w477, "variant"=w478) -> (w479:T9)
              n168 = Build Array(w473) -> (w481:T4[])
              n169 = Build Array(w479) -> (w476:T15)
            }
          }
        }
        frame "Intersection(Search)" {
          n170 = Unbundle By Name(w497) -> ("Type A"=w517:enum16{"Curves", "Values", "Results", "WFM"}, "Type B"=w514:enum16{"Curves", "Values", "Results", "WFM"}, "Custom unit info"=w529:T16, "Search Items"=w493:string[], "All points"=w492:bool, "Search Mode"=w510:u16)
          n171 = Index Array(array=w502) -> (element=w501:T2)  [unwired: 1 in]
          n172 = Unbundle By Name(w501) -> ("Res Name"=w499:string)
          n173 = Not Equal?(x=w517, y=enum16{"Curves", "Values", "Results", "WFM"}."WFM" ("Type A")) -> (x != y?=w524:bool)
          n174 = Not Equal?(x=w514, y=enum16{"Curves", "Values", "Results", "WFM"}."WFM" ("Type A")) -> (x != y?=w521:bool)
          n175 = Not(x=w524) -> (.not. x?=w523:bool)
          n176 = Not(x=w521) -> (.not. x?=w522:bool)
          n177 = And(x=w524, y=w522) -> (x .and. y?=w520:bool)
          n178 = And(x=w524, y=w521) -> (x .and. y?=w527:bool)
          n179 = And(x=w523, y=w521) -> (x .and. y?=w519:bool)
          n180 = And(x=w523, y=w522) -> (x .and. y?=w518:bool)
          n181 = Build Array(w527, w520, w519, w518) -> (w526:bool[])
          n182 = Search 1D Array(1D array=w526, element=TRUE) -> (index of element=w513:i32)  [unwired: 1 out]
          n183 = case shown="1, 2" w513 {
            tunnel: w530 -> [w550 w555 _]
            tunnel: w528 -> [w551 _ _]
            tunnel: [w549 w554 w556] -> w491
            tunnel: w512 -> [_ _ w560]
            tunnel: w511 -> [_ _ w561]
            tunnel: w493 -> [w548 _ w558]
            tunnel: w492 -> [w547 _ w557]
            frame 0, Default {
              n184 = call "CRYSearch for Intersection.vi"("All points"=w547, "Search range"=w548, "Supress warnings (F)"=TRUE, "Operand B"=w551, "Operand A"=w550) -> ("Resulting data"=w549:T4)  [unwired: 6 out]
            }
            frame 1, 2 {
              n185 = Bundle By Name(cluster=w555, "Curve"=cluster{"x":dbl, "y":dbl, "z":dbl}[] [{"x"=nan, "y"=nan, "z"=nan}]) -> (w554:T4)
            }
            frame 3 {
              n186 = call "CRYSearch for Intersection of Wave.vi"("All points"=w557, "Search range"=w558, "Supress warnings (F)"=TRUE, "Waveform B"=w560, "Waveform A"=w561) -> ("Resulting data"=w556:T4)  [unwired: 6 in]
            }
          }
          n187 = case shown="0, Default" w510 {
            tunnel: w491 -> [w534 w541 w546]
            tunnel: [w532 w537 w544] -> w488
            frame 0, Default {
              n188 = Unbundle By Name(w534) -> ("Curve"=w536:cluster{"x":dbl, "y":dbl, "z":dbl}[])
              n189 = Index Array(array=w536) -> (element=w535:cluster{"x":dbl, "y":dbl, "z":dbl})  [unwired: 1 in]
              n190 = Build Array(w535) -> (w533:cluster{"x":dbl, "y":dbl, "z":dbl}[])
              n191 = Bundle By Name(cluster=w534, "single val"=TRUE, "Curve"=w533) -> (w532:T4)
            }
            frame 1 {
              n192 = Unbundle By Name(w541) -> ("Curve"=w543:cluster{"x":dbl, "y":dbl, "z":dbl}[])
              n193 = Reverse 1D Array(array=w543) -> (reversed array=w542:cluster{"x":dbl, "y":dbl, "z":dbl}[])
              n194 = Index Array(array=w542) -> (element=w540:cluster{"x":dbl, "y":dbl, "z":dbl})  [unwired: 1 in]
              n195 = Build Array(w540) -> (w539:cluster{"x":dbl, "y":dbl, "z":dbl}[])
              n196 = Bundle By Name(cluster=w541, "single val"=TRUE, "Curve"=w539) -> (w537:T4)
            }
            frame 2 {
              n197 = Bundle By Name(cluster=w546, "single val"=FALSE) -> (w544:T4)
            }
          }
          n198 = Unbundle By Name(w497) -> ("x"=w496:bool, "y"=w495:bool, "z"=w494:bool)
          n199 = Unbundle By Name(w488) -> ("Y unit"=w489:string)
          n200 = call "CRYCustom Unit Convert.vi"("Custom unit info"=w529, "Axis Mode"=u16 1, "Data in"=w488) -> ("Data out"=w500:T4)  [unwired: 8 out]
          n201 = Bundle By Name(cluster=w500, "Name"=w499, "display X"=w496, "display Y"=w495, "display Z"=w494) -> (w498:T4)
          n202 = call "CRYSpiltOnlyUnit.vi"("In Unit String"=w489) -> ("Out Unit String"=w490:string)  [unwired: 10 in]
          n203 = global write "CRYPost Processing Global.vi" "disp_unit"(w490) -> ()
          n204 = To Variant(anything=w498) -> (Variant=w506:variant)
          n205 = Bundle By Name(cluster=w503, "variant"=w506) -> (w505:T9)
          n206 = Build Array(w498) -> (w508:T4[])
          n207 = Build Array(w505) -> (w504:T15)
        }
        frame "User Equation" {
          n208 = global read "CRYMainGlobal.vi" "top path"() -> (w568:path)
          n209 = Build Path(base path=w568, name or relative path="CRYSystem\\Post Processing\\SubVI\\CRYUser Equation Parametes Table.vi" ("StepName")) -> (appended path=w570:path)
          n210 = Open VI Reference(vi path=w570) -> (vi reference=w565:refnum<vi>, error out=w564:errorcluster)  [unwired: 1 in, 4 out]
          n211 = property class="VI"(reference=w565, error in=w564) -> ("Front Panel.Open"=w566:bool)  [unwired: 2 out]
          n212 = stacked-sequence {
            tunnel: w563 -> [w586 _]
            tunnel: [w580 _] -> w573
            tunnel: w566 -> [w582 w597]
            tunnel: w563 -> [w579 _]
            tunnel: w562 -> [w578 _]
            frame #0 {
              n213 = Unbundle By Name(w586) -> ("user equation cluster"=w585:T12)
              n214 = call "CRYCalculate User Equation.vi"("No.VI"=w578, "User equation cluster In"=w585) -> ("Result Curves"=w581:T4[], "User equation cluster Out"=w584:T12)  [unwired: 7 in, 1 out]
              n215 = call "CRYFlatten User Equation Cluster.vi"("user equation cluster"=w584) -> ("Flatten String"=w583:string)  [unwired: 10 in]
              n216 = case shown="True" w582 {
                tunnel: w583 -> [_ w593]
                frame False {
                }
                frame True {
                  n217 = global read "CRYPost Processing Global.vi" "Post Editor VI Ref"() -> (w595:refnum<vi>)
                  n218 = call "CRYGet String Reference.vi"("Label Name"="User Equation String", "VI Refnum"=w595) -> ("String Ref Out"=w594:refnum<vi>)  [unwired: 9 out]
                  n219 = property class="Str"(reference=w594, "Val(Sgnl)"=w593) -> ()  [unwired: 1 in, 2 out]
                }
              }
              n220 = for {
                tunnel: w581 -> [w592] mode=indexing
                tunnel: [w591] -> w580 mode=indexing
                tunnel: w579 -> [w590]
                n221 = Unbundle By Name(w590) -> ("x"=w589:bool, "y"=w588:bool, "z"=w587:bool)
                n222 = Bundle By Name(cluster=w592, "display X"=w589, "display Y"=w588, "display Z"=w587) -> (w591:T4)
              }
            }
            frame #1 {
              n223 = case shown="True" w597 {
                frame False {
                }
                frame True {
                  n224 = global read "CRYPost Processing Global.vi" "User Equation VI Ref"() -> (w598:refnum<vi>)
                  n225 = call "CRYGet Boolean Reference.vi"("Label Name"=" Res_Table Change", "VI Refnum"=w598) -> ("Boolean Ref"=w600:refnum<vi>)  [unwired: 7 in, 2 out]
                  n226 = property class="Bool"(reference=w600, "Val(Sgnl)"=TRUE) -> ()  [unwired: 1 in, 2 out]
                }
              }
            }
          }
          n227 = for {
            tunnel: w573 -> [w576] mode=indexing
            tunnel: w572 -> [w575]
            tunnel: [w574] -> w571 mode=indexing
            n228 = To Variant(anything=w576) -> (Variant=w577:variant)
            n229 = Bundle By Name(cluster=w575, "variant"=w577) -> (w574:T9)
          }
        }
        frame "Windowing" {
          n230 = Unbundle By Name(w620) -> ("Custom unit info"=w615:T16, "Type A"=w612:enum16{"Curves", "Values", "Results", "WFM"}, "Search Items"=w618:string[], "All points"=w619:bool, "x"=w604:bool, "y"=w603:bool, "z"=w602:bool)
          n231 = Index Array(array=w607) -> (element=w606:T2)  [unwired: 1 in]
          n232 = Unbundle By Name(w606) -> ("Res Name"=w605:string)
          n233 = case shown="True" w619 {
            tunnel: w612 -> [w635 w692]
            tunnel: w617 -> [w634 w696]
            tunnel: w616 -> [w633 w695]
            tunnel: w618 -> [w632 _]
            tunnel: [w631 w694] -> w610
            tunnel: [w630 w693] -> w611
            tunnel: w615 -> [w629 w691]
            tunnel: w614 -> [w628 w690]
            tunnel: w613 -> [w627 w689]
            tunnel: w609 -> [w626 w688]
            tunnel: [w625 w687] -> w608
            tunnel: w605 -> [w624 w686]
            tunnel: w604 -> [w623 w685]
            tunnel: w603 -> [w622 w684]
            tunnel: w602 -> [w621 w683]
            frame False {
              n234 = case shown="\"Curves\", Default" w635 {
                tunnel: w634 -> [w655 _]
                tunnel: w633 -> [_ w675]
                tunnel: w632 -> [w658 w678]
                tunnel: [w649 w672] -> w631
                tunnel: [w650 w671] -> w630
                tunnel: w629 -> [w652 _]
                tunnel: w628 -> [w649 _]
                tunnel: w627 -> [_ w671]
                tunnel: w626 -> [w646 w668]
                tunnel: [w645 w667] -> w625
                tunnel: w624 -> [w643 w666]
                tunnel: w623 -> [w641 w664]
                tunnel: w622 -> [w640 w663]
                tunnel: w621 -> [w639 _]
                frame "Curves", Default {
                  n235 = Unbundle By Name(w655) -> ("Curve"=w659:cluster{"x":dbl, "y":dbl, "z":dbl}[], "X axis"=w657:u16)
                  n236 = Sort 1D Array(array=w659) -> (sorted array=w653:cluster{"x":dbl, "y":dbl, "z":dbl}[])
                  n237 = call "CRYCurve Cut to Range.vi"("Axis type (Lin)"=w657, "Range variable (x)"=enum16{"x", "y", "z"}."x", "Search range"=w658, "Curve in"=w653) -> ("Cut curve out"=w656:cluster{"x":dbl, "y":dbl, "z":dbl}[])  [unwired: 7 out]
                  n238 = Bundle By Name(cluster=w655, "Curve"=w656) -> (w636:T4)
                  n239 = call "CRYCustom Unit Convert.vi"("Custom unit info"=w652, "Axis Mode"=u16 1, "Data in"=w636) -> ("Data out"=w644:T4)  [unwired: 8 out]
                  n240 = Bundle By Name(cluster=w644, "Name"=w643, "display X"=w641, "display Y"=w640, "display Z"=w639) -> (w642:T4)
                  n241 = Unbundle By Name(w636) -> ("Y unit"=w637:string)
                  n242 = call "CRYSpiltOnlyUnit.vi"("In Unit String"=w637) -> ("Out Unit String"=w638:string)  [unwired: 10 in]
                  n243 = global write "CRYPost Processing Global.vi" "disp_unit"(w638) -> ()
                  n244 = To Variant(anything=w642) -> (Variant=w648:variant)
                  n245 = Bundle By Name(cluster=w646, "variant"=w648) -> (w647:T9)
                  n246 = Build Array(w642) -> (w650:T4[])
                  n247 = Build Array(w647) -> (w645:T15)
                }
                frame "WFM" {
                  n248 = call "CRYWaveform to DAT.vi"("Waveform In"=w675) -> ("Curve Out"=w676:T4)  [unwired: 10 out]
                  n249 = Unbundle By Name(w676) -> ("Curve"=w682:cluster{"x":dbl, "y":dbl, "z":dbl}[], "X axis"=w681:u16)
                  n250 = Sort 1D Array(array=w682) -> (sorted array=w673:cluster{"x":dbl, "y":dbl, "z":dbl}[])
                  n251 = Unbundle By Name(w675) -> ("Waveform.dX"=w674:dbl)
                  n252 = call "CRYCurve Cut to Range.vi"("Axis type (Lin)"=w681, "Range variable (x)"=enum16{"x", "y", "z"}."x", "Search range"=w678, "Curve in"=w673) -> ("Cut curve out"=w680:cluster{"x":dbl, "y":dbl, "z":dbl}[])  [unwired: 7 out]
                  n253 = Bundle By Name(cluster=w676, "Curve"=w680) -> (w677:T4)
                  n254 = call "CRYDAT to Waveform.vi"("dX"=w674, "Curve In"=w677) -> ("Waveform Out"=w660:T8)  [unwired: 9 out]
                  n255 = Bundle By Name(cluster=w660, "Name"=w666, "display X"=w664, "display Y"=w663) -> (w665:T8)
                  n256 = Unbundle By Name(w660) -> ("Y unit"=w661:string)
                  n257 = To Variant(anything=w665) -> (Variant=w670:variant)
                  n258 = call "CRYSpiltOnlyUnit.vi"("In Unit String"=w661) -> ("Out Unit String"=w662:string)  [unwired: 10 in]
                  n259 = Bundle By Name(cluster=w668, "variant"=w670) -> (w669:T9)
                  n260 = global write "CRYPost Processing Global.vi" "disp_unit"(w662) -> ()
                  n261 = Build Array(w665) -> (w672:T8[])
                  n262 = Build Array(w669) -> (w667:T15)
                }
              }
            }
            frame True {
              n263 = case shown="\"WFM\"" w692 {
                tunnel: w696 -> [w697 _]
                tunnel: w695 -> [_ w715]
                tunnel: [w710 w725] -> w694
                tunnel: [w711 w726] -> w693
                tunnel: w691 -> [w713 _]
                tunnel: w690 -> [w710 _]
                tunnel: w689 -> [_ w726]
                tunnel: w688 -> [w707 w722]
                tunnel: [w706 w721] -> w687
                tunnel: w686 -> [w704 w720]
                tunnel: w685 -> [w702 w719]
                tunnel: w684 -> [w701 w718]
                tunnel: w683 -> [w700 _]
                frame "Curves", Default {
                  n264 = call "CRYCustom Unit Convert.vi"("Custom unit info"=w713, "Axis Mode"=u16 1, "Data in"=w697) -> ("Data out"=w705:T4)  [unwired: 8 out]
                  n265 = Unbundle By Name(w697) -> ("Y unit"=w698:string)
                  n266 = Bundle By Name(cluster=w705, "Name"=w704, "display X"=w702, "display Y"=w701, "display Z"=w700) -> (w703:T4)
                  n267 = call "CRYSpiltOnlyUnit.vi"("In Unit String"=w698) -> ("Out Unit String"=w699:string)  [unwired: 10 in]
                  n268 = global write "CRYPost Processing Global.vi" "disp_unit"(w699) -> ()
                  n269 = To Variant(anything=w703) -> (Variant=w709:variant)
                  n270 = Bundle By Name(cluster=w707, "variant"=w709) -> (w708:T9)
                  n271 = Build Array(w703) -> (w711:T4[])
                  n272 = Build Array(w708) -> (w706:T15)
                }
                frame "WFM" {
                  n273 = Bundle By Name(cluster=w715, "Name"=w720, "display X"=w719, "display Y"=w718) -> (w714:T8)
                  n274 = Unbundle By Name(w714) -> ("Y unit"=w716:string)
                  n275 = To Variant(anything=w714) -> (Variant=w724:variant)
                  n276 = call "CRYSpiltOnlyUnit.vi"("In Unit String"=w716) -> ("Out Unit String"=w717:string)  [unwired: 10 in]
                  n277 = Build Array(w714) -> (w725:T8[])
                  n278 = Bundle By Name(cluster=w722, "variant"=w724) -> (w723:T9)
                  n279 = global write "CRYPost Processing Global.vi" "disp_unit"(w717) -> ()
                  n280 = Build Array(w723) -> (w721:T15)
                }
              }
            }
          }
        }
        frame "Resolution" {
          n281 = Unbundle By Name(w751) -> ("New Resolution"=w750:u16, "Freq Mode"=w749:u16, "Hz"=w748:dbl, "Custom unit info"=w746:T16, "x"=w734:bool, "y"=w733:bool, "z"=w732:bool)
          n282 = Index Array(array=w739) -> (element=w738:T2)  [unwired: 1 in]
          n283 = Unbundle By Name(w738) -> ("Res Name"=w736:string)
          n284 = call "CRYCurve Resolution.vi"("smoothing"=w727, "1/nOct_Hz"=w748, "Frequencies"=w749, "New Resolution"=w750, "Curve in"=w728) -> ("Curve out"=w729:T4)  [unwired: 6 out]
          n285 = call "CRYCustom Unit Convert.vi"("Custom unit info"=w746, "Axis Mode"=u16 1, "Data in"=w729) -> ("Data out"=w737:T4)  [unwired: 8 out]
          n286 = Unbundle By Name(w729) -> ("Y unit"=w730:string)
          n287 = Bundle By Name(cluster=w737, "Name"=w736, "display X"=w734, "display Y"=w733, "display Z"=w732) -> (w735:T4)
          n288 = call "CRYSpiltOnlyUnit.vi"("In Unit String"=w730) -> ("Out Unit String"=w731:string)  [unwired: 10 in]
          n289 = global write "CRYPost Processing Global.vi" "disp_unit"(w731) -> ()
          n290 = Build Array(w735) -> (w745:T4[])
          n291 = To Variant(anything=w735) -> (Variant=w743:variant)
          n292 = Bundle By Name(cluster=w741, "variant"=w743) -> (w742:T9)
          n293 = Build Array(w742) -> (w740:T15)
        }
        frame "Directivity Index" {
          n294 = Unbundle By Name(w777) -> ("Curve Group"=w754:string[], "Custom unit info"=w775:T16, "x"=w763:bool, "y"=w762:bool, "z"=w761:bool, "Weighting Curve"=w758:string, "Direct Weighting"=w759:bool, "Auto Inc"=w753:bool, "Inc(deg)"=w756:i32, "Total Rotation"=w752:i32)
          n295 = Index Array(array=w767) -> (element=w768:T2)  [unwired: 1 in]
          n296 = Unbundle By Name(w768) -> ("Res Name"=w765:string)
          n297 = call "CRYCalc Directivity Index.vi"("Weighting curve"=w758, "Direct_weight"=w759, "Inc(deg.)"=w756, "Total Rotation"=w752, "Curve Group"=w754, "Auto Inc"=w753, "Curve in"=w755) -> ("Curve out"=w757:T4)  [unwired: 4 out]
          n298 = call "CRYCustom Unit Convert.vi"("Custom unit info"=w775, "Axis Mode"=u16 1, "Data in"=w757) -> ("Data out"=w766:T4)  [unwired: 8 out]
          n299 = Bundle By Name(cluster=w766, "Name"=w765, "display X"=w763, "display Y"=w762, "display Z"=w761) -> (w764:T4)
          n300 = global write "CRYPost Processing Global.vi" "disp_unit"("") -> ()
          n301 = To Variant(anything=w764) -> (Variant=w772:variant)
          n302 = Build Array(w764) -> (w774:T4[])
          n303 = Bundle By Name(cluster=w770, "variant"=w772) -> (w771:T9)
          n304 = Build Array(w771) -> (w769:T15)
        }
        frame "1/n Octave Synthesis" {
          n305 = Unbundle By Name(w799) -> ("New Resolution"=w798:u16, "Custom unit info"=w796:T16, "x"=w783:bool, "y"=w782:bool, "z"=w781:bool)
          n306 = Index Array(array=w787) -> (element=w788:T2)  [unwired: 1 in]
          n307 = Unbundle By Name(w788) -> ("Res Name"=w785:string)
          n308 = call "CRYOctave synthesis.vi"("New Resolution"=w798, "Curve in"=w797) -> ("Curve out"=w778:T4)  [unwired: 1 in, 8 out]
          n309 = Unbundle By Name(w778) -> ("Y unit"=w779:string)
          n310 = call "CRYCustom Unit Convert.vi"("Custom unit info"=w796, "Axis Mode"=u16 1, "Data in"=w778) -> ("Data out"=w786:T4)  [unwired: 8 out]
          n311 = Bundle By Name(cluster=w786, "Name"=w785, "display X"=w783, "display Y"=w782, "display Z"=w781) -> (w784:T4)
          n312 = call "CRYSpiltOnlyUnit.vi"("In Unit String"=w779) -> ("Out Unit String"=w780:string)  [unwired: 10 in]
          n313 = global write "CRYPost Processing Global.vi" "disp_unit"(w780) -> ()
          n314 = Build Array(w784) -> (w794:T4[])
          n315 = To Variant(anything=w784) -> (Variant=w792:variant)
          n316 = Bundle By Name(cluster=w790, "variant"=w792) -> (w791:T9)
          n317 = Build Array(w791) -> (w789:T15)
        }
        frame "Resampling" {
          n318 = Unbundle By Name(w811) -> ("Name"=w810:string, "Waveform.Y"=w806:sgl[])
          n319 = Index Array(array=w813) -> (element=w814:T2)  [unwired: 1 in]
          n320 = Unbundle By Name(w814) -> ("Res Name"=w812:string)
          n321 = Empty String/Path?(string/path=w810) -> (empty?=w804:bool)
          n322 = Array Size(array=w806) -> (size(s)=w807:i32)
          n323 = Equal To 0?(x=w807) -> (x = 0?=w808:bool)
          n324 = Or(x=w804, y=w808) -> (x .or. y?=w805:bool)
          n325 = case shown="True" w805 {
            tunnel: w818 -> [w831 _]
            tunnel: [w830 w837] -> w801
            tunnel: w816 -> [w827 w834]
            tunnel: [w825 w836] -> w815
            tunnel: w812 -> [w824 w832]
            tunnel: w811 -> [w823 w833]
            tunnel: w809 -> [_ w837]
            tunnel: w804 -> [_ w835]
            frame False {
              n326 = Unbundle By Name(w831) -> ("y"=w822:bool, "x"=w821:bool, "New Sampling Rate"=w820:dbl)
              n327 = call "CRYWaveform Resampling.vi"("New Sampling Rate"=w820, "Wave"=w823) -> ("New Wave"=w819:T8)  [unwired: 9 in]
              n328 = Bundle By Name(cluster=w819, "display Y"=w822, "display X"=w821, "Name"=w824) -> (w826:T8)
              n329 = To Variant(anything=w826) -> (Variant=w829:variant)
              n330 = Bundle By Name(cluster=w827, "variant"=w829) -> (w828:T9)
              n331 = Build Array(w826) -> (w830:T8[])
              n332 = Build Array(w828) -> (w825:T15)
            }
            frame True {
              n333 = case shown="False" w835 {
                tunnel: [w842 T15 []] -> w836
                tunnel: w834 -> [w843 _]
                tunnel: w833 -> [w841 _]
                tunnel: w832 -> [w840 _]
                frame False {
                  w838 = TRUE ("display Y")
                  n334 = Bundle By Name(cluster=w841, "display Y"=w838, "display X"=w838, "Name"=w840) -> (w839:T8)
                  n335 = To Variant(anything=w839) -> (Variant=w845:variant)
                  n336 = Bundle By Name(cluster=w843, "variant"=w845) -> (w844:T9)
                  n337 = Build Array(w844) -> (w842:T15)
                }
                frame True {
                }
              }
            }
          }
          n338 = Index Array(array=w801) -> (element=w800:T8)  [unwired: 1 in]
          n339 = Unbundle By Name(w800) -> ("Y unit"=w802:string)
          n340 = call "CRYSpiltOnlyUnit.vi"("In Unit String"=w802) -> ("Out Unit String"=w803:string)  [unwired: 10 in]
          n341 = global write "CRYPost Processing Global.vi" "disp_unit"(w803) -> ()
        }
        frame "Frequency Shift" {
          # "++result=Playback sampling rate(Single Value)=zhunque ?"
          n342 = Unbundle By Name(w853) -> ("Name"=w869:string, "Waveform.Y"=w866:sgl[])
          n343 = Index Array(array=w857, index #1=0 ("index"), index #2=1 ("index")) -> (element #1=w858:T2, element #2=w861:T2)
          n344 = Empty String/Path?(string/path=w869) -> (empty?=w862:bool)
          n345 = Array Size(array=w866) -> (size(s)=w865:i32)
          n346 = Unbundle By Name(w861) -> ("Res Name"=w855:string)
          n347 = Unbundle By Name(w858) -> ("Res Name"=w856:string)
          n348 = Equal To 0?(x=w865) -> (x = 0?=w864:bool)
          n349 = Or(x=w862, y=w864) -> (x .or. y?=w863:bool)
          n350 = call "CRYUnflatten Data.vi"() -> ("Datum"=w854:T4)  [unwired: 9 in, 2 out]
          n351 = case shown="False" w863 {
            tunnel: w873 -> [w885 _]
            tunnel: [w884 w958] -> w872
            tunnel: [w883 w957] -> w850
            tunnel: w871 -> [w882 w952]
            tunnel: [w881 w962] -> w870
            tunnel: w868 -> [_ w960]
            tunnel: w867 -> [_ w959]
            tunnel: w862 -> [_ w961]
            tunnel: w856 -> [w880 w955]
            tunnel: w855 -> [w879 w954]
            tunnel: w854 -> [w878 w953]
            tunnel: w853 -> [w877 w956]
            tunnel: w848 -> [w874 _]
            tunnel: w847 -> [w875 _]
            frame False {
              n352 = Equal To 0?(x=w874) -> (x = 0?=w876:bool)
              n353 = case shown="True" w876 {
                tunnel: w885 -> [w889 w949]
                tunnel: [w894 w942] -> w884
                tunnel: [w893 w941] -> w883
                tunnel: w882 -> [w896 w937]
                tunnel: [w895 w935] -> w881
                tunnel: w880 -> [w892 w928]
                tunnel: w879 -> [w891 w927]
                tunnel: w878 -> [w897 w926]
                tunnel: w877 -> [w890 w925]
                tunnel: w875 -> [w888 w921]
                tunnel: w874 -> [w887 w920]
                frame False {
                  w902 = TRUE ("display Y")
                  w901 = FALSE ("display Y")
                  n354 = Unbundle By Name(w889) -> ("Ref Freq Mode"=w911:u16, "Ref Waveform"=w910:string, "Ref Freq"=w912:dbl)
                  n355 = case shown="0, Default" w911 {
                    tunnel: w910 -> [w917 _]
                    tunnel: [w917 ""] -> w899
                    frame 0, Default {
                    }
                    frame 1 {
                    }
                  }
                  n356 = call "CRYFrequency Shift.vi"("User Sampling Rate"=w888, "Freq Sampling Mode"=w887, "Reference Frequency"=w912, "Source Wave Name"=w899, "Waveform In"=w890) -> ("PlaybackSamplingRate"=w886:dbl, "Wave Out"=w904:T8)  [unwired: 5 in]
                  n357 = Bundle By Name(cluster=cluster{"x":dbl, "y":dbl, "z":dbl} {"x"=0.0, "y"=0.0, "z"=0.0}, "x"=w886) -> (w915:cluster{"x":dbl, "y":dbl, "z":dbl})
                  n358 = Build Array(w915) -> (w914:cluster{"x":dbl, "y":dbl, "z":dbl}[])
                  n359 = Bundle By Name(cluster=w897, "Curve"=w914, "single val"=TRUE, "Name"=w892, "display X"=TRUE, "display Y"=w901, "display Z"=w901, "X unit"="Hz") -> (w905:T4)
                  n360 = Bundle By Name(cluster=w904, "Name"=w891, "display X"=w902, "display Y"=w902) -> (w898:T8)
                  n361 = To Variant(anything=w905) -> (Variant=w908:variant)
                  n362 = To Variant(anything=w898) -> (Variant=w909:variant)
                  n363 = Bundle By Name(cluster=w896, "variant"=w908) -> (w907:T9)
                  n364 = Bundle By Name(cluster=w896, "variant"=w909) -> (w906:T9)
                  n365 = Build Array(w907, w906) -> (w895:T15)
                  n366 = Build Array(w905) -> (w894:T4[])
                  n367 = Build Array(w898) -> (w893:T8[])
                }
                frame True {
                  w931 = TRUE ("display Y")
                  w930 = FALSE ("display Y")
                  n368 = Unbundle By Name(w949) -> ("Ref Freq Mode"=w919:u16, "Ref Waveform"=w943:string, "Ref Freq"=w944:dbl)
                  n369 = case shown="1" w919 {
                    tunnel: w943 -> [w950 _]
                    tunnel: [w950 ""] -> w924
                    frame 0, Default {
                    }
                    frame 1 {
                    }
                  }
                  n370 = call "CRYFrequency Shift.vi"("User Sampling Rate"=w921, "Freq Sampling Mode"=w920, "Reference Frequency"=w944, "Source Wave Name"=w924, "Waveform In"=w925) -> ("PlaybackSamplingRate"=w923:dbl, "Wave Out"=w933:T8)  [unwired: 5 in]
                  n371 = Bundle By Name(cluster=cluster{"x":dbl, "y":dbl, "z":dbl} {"x"=0.0, "y"=0.0, "z"=0.0}, "x"=w923) -> (w947:cluster{"x":dbl, "y":dbl, "z":dbl})
                  n372 = Build Array(w947) -> (w946:cluster{"x":dbl, "y":dbl, "z":dbl}[])
                  n373 = Bundle By Name(cluster=w926, "Curve"=w946, "single val"=TRUE, "Name"=w928, "display X"=TRUE, "display Y"=w930, "display Z"=w930, "X unit"="Hz") -> (w934:T4)
                  n374 = Bundle By Name(cluster=w933, "Name"=w927, "display X"=w931, "display Y"=w931) -> (w922:T8)
                  n375 = To Variant(anything=w934) -> (Variant=w939:variant)
                  n376 = To Variant(anything=w922) -> (Variant=w940:variant)
                  n377 = Bundle By Name(cluster=w937, "variant"=w939) -> (w938:T9)
                  n378 = Bundle By Name(cluster=w937, "variant"=w940) -> (w936:T9)
                  n379 = Build Array(w938, w936) -> (w935:T15)
                  n380 = Build Array(w934) -> (w942:T4[])
                  n381 = Build Array(w922) -> (w941:T8[])
                }
              }
            }
            frame True {
              n382 = case shown="True" w961 {
                tunnel: [w967 T15 []] -> w962
                tunnel: w960 -> [_ w982]
                tunnel: w959 -> [_ w981]
                tunnel: [w965 w982] -> w958
                tunnel: [w963 w981] -> w957
                tunnel: w956 -> [w974 _]
                tunnel: w955 -> [w976 _]
                tunnel: w954 -> [w973 _]
                tunnel: w953 -> [w978 _]
                tunnel: w952 -> [w968 _]
                frame False {
                  w975 = TRUE ("display Y")
                  w980 = FALSE ("display Y")
                  w977 = TRUE ("display X")
                  n383 = Bundle By Name(cluster=w978, "single val"=w977, "Name"=w976, "display X"=w977, "display Y"=w980, "display Z"=w980, "X unit"="Hz") -> (w966:T4)
                  n384 = Bundle By Name(cluster=w974, "Name"=w973, "display X"=w975, "display Y"=w975) -> (w964:T8)
                  n385 = To Variant(anything=w966) -> (Variant=w971:variant)
                  n386 = To Variant(anything=w964) -> (Variant=w972:variant)
                  n387 = Bundle By Name(cluster=w968, "variant"=w971) -> (w970:T9)
                  n388 = Bundle By Name(cluster=w968, "variant"=w972) -> (w969:T9)
                  n389 = Build Array(w966) -> (w965:T4[])
                  n390 = Build Array(w964) -> (w963:T8[])
                  n391 = Build Array(w970, w969) -> (w967:T15)
                }
                frame True {
                }
              }
            }
          }
          n392 = Index Array(array=w850) -> (element=w849:T8)  [unwired: 1 in]
          n393 = Unbundle By Name(w849) -> ("Y unit"=w851:string)
          n394 = call "CRYSpiltOnlyUnit.vi"("In Unit String"=w851) -> ("Out Unit String"=w852:string)  [unwired: 10 in]
          n395 = global write "CRYPost Processing Global.vi" "disp_unit"(w852) -> ()
        }
        frame "Boolean" {
          n396 = Index Array(array=w987) -> (element=w986:T2)  [unwired: 1 in]
          n397 = for {
            tunnel: enum16{"Curves", "Values", "Results", "WFM"}."Results" ("Type") -> [w1002]
            tunnel: w990 -> [w1001] mode=indexing
            tunnel: [w999] -> w989 mode=indexing
            n398 = call "CRYGet Curve Library One Data .vi"("Data Name"=w1001, "Type"=w1002) -> ("Result"=w1000:T6)  [unwired: 3 in, 6 out]
            n399 = Unbundle By Name(w1000) -> ("Verdict"=w999:bool)
          }
          n400 = Unbundle By Name(w986) -> ("Res Name"=w985:string)
          n401 = And Array Elements(Boolean array=w989) -> (logical AND=w988:bool)
          n402 = call "CRYUnflatten Results.vi"() -> ("Result"=w996:T6)  [unwired: 9 in, 2 out]
          n403 = Bundle By Name(cluster=w996, "Name"=w985, "Verdict"=w988, "Margin"=0.0) -> (w993:T6)
          n404 = To Variant(anything=w993) -> (Variant=w995:variant)
          n405 = Bundle By Name(cluster=w998, "variant"=w995) -> (w994:T9)
          n406 = Build Array(w994) -> (w997:T15)
          n407 = Build Array(w993) -> (w992:T6[])
        }
      }
      "Result Out" <- w117
      "Data out" <- w135
      "Wave out" <- w134
      n408 = for {
        tunnel: w132 -> [w1015] mode=indexing
        tunnel: w127 -> [w1014]
        tunnel: w131 -> [w1013] mode=indexing
        shift-right: [w1009] -> w128
        shift-left: w125 -> [w1010]
        shift-right: [w1007] -> w129
        shift-left: w126 -> [w1008]
        shift-right: [w1005] -> w130
        shift-left: w126 -> [w1006]
        shift-right: [w1003] -> w119
        shift-left: w116 -> [w1004]
        n409 = Unbundle By Name(w1013) -> ("Type out"=w1011:enum16{"Curves", "Values", "Results", "WFM"}, "Res Name"=w1012:string)
        n410 = case shown="\"Results\"" w1011 {
          tunnel: w1015 -> [w1027 w1047 w1059]
          tunnel: w1014 -> [w1025 w1049 w1061]
          tunnel: w1012 -> [w1026 w1048 w1060]
          tunnel: w1010 -> [w1020 w1043 w1050]
          tunnel: [w1020 w1042 w1050] -> w1009
          tunnel: w1008 -> [w1022 w1041 w1055]
          tunnel: [w1021 w1041 w1055] -> w1007
          tunnel: w1006 -> [w1019 w1040 w1054]
          tunnel: [w1018 w1040 w1054] -> w1005
          tunnel: w1004 -> [w1016 w1038 w1052]
          tunnel: [w1016 w1038 w1051] -> w1003
          frame "Curves", "Values", Default {
            n411 = Unbundle By Name(w1027) -> ("variant"=w1028:variant)
            n412 = call "CRYUnflatten Data.vi"() -> ("Datum"=w1029:T4)  [unwired: 9 in, 2 out]
            n413 = Variant To Data(type=w1029, Variant=w1028) -> (data=w1024:T4)  [unwired: 1 in, 1 out]
            n414 = Bundle By Name(cluster=w1024, "Name"=w1026, "Step No."=w1025) -> (w1017:T4)
            n415 = Unbundle By Name(w1024) -> ("single val"=w1023:bool)
            n416 = case shown="True" w1023 {
              tunnel: w1017 -> [w1032 w1037]
              tunnel: w1022 -> [w1033 w1036]
              tunnel: [w1033 w1035] -> w1021
              tunnel: w1019 -> [w1031 w1034]
              tunnel: [w1030 w1034] -> w1018
              frame False {
                n417 = Insert Into Array(array=w1031, new element=w1032) -> (w1030:T4[])  [unwired: 1 in]
              }
              frame True {
                n418 = Insert Into Array(array=w1036, new element=w1037) -> (w1035:T4[])  [unwired: 1 in]
              }
            }
          }
          frame "WFM" {
            n419 = Unbundle By Name(w1047) -> ("variant"=w1046:variant)
            n420 = call "CRYUnFlatten waveform.vi"() -> ("Waveform Cluster"=w1045:T8)  [unwired: 9 in, 2 out]
            n421 = Variant To Data(type=w1045, Variant=w1046) -> (data=w1044:T8)  [unwired: 1 in, 1 out]
            n422 = Bundle By Name(cluster=w1044, "Name"=w1048, "Step No."=w1049) -> (w1039:T8)
            n423 = Insert Into Array(array=w1043, new element=w1039) -> (w1042:T8[])  [unwired: 1 in]
          }
          frame "Results" {
            n424 = Unbundle By Name(w1059) -> ("variant"=w1058:variant)
            n425 = call "CRYUnflatten Results.vi"() -> ("Result"=w1057:T6)  [unwired: 9 in, 2 out]
            n426 = Variant To Data(type=w1057, Variant=w1058) -> (data=w1056:T6)  [unwired: 1 in, 1 out]
            n427 = Bundle By Name(cluster=w1056, "Name"=w1060, "Step No."=w1061) -> (w1053:T6)
            n428 = Insert Into Array(array=w1052, new element=w1053) -> (w1051:T6[])  [unwired: 1 in]
          }
        }
      }
    }
  }
  n429 = Index Array(array=w28, index=1) -> (element=w19:bool)
  n430 = global read "CRYProject Run Control Global.vi" "RunState"() -> (w17:bool)
  n431 = Select(t="Overwrite" ("Y unit"), s=w19, f="Repeat") -> (s? t:f=w27:string)
  n432 = case shown="False" w17 {
    tunnel: ["Apply" ("sOption1") "Run" ("Type In")] -> w16
    tunnel: ["APPLY_CURVE" ("Type In") "RUN_CURVE" ("Type In")] -> w15
    frame False {
    }
    frame True {
    }
  }
  n433 = case shown="False" w19 {
    tunnel: w22 -> [w1075 w1079]
    tunnel: w21 -> [w1074 w1078]
    tunnel: w20 -> [w1073 w1077]
    tunnel: [w1072 w1079] -> w13
    tunnel: [w1071 w1078] -> w12
    tunnel: [w1070 w1077] -> w11
    tunnel: w18 -> [w1069 _]
    tunnel: w15 -> [w1068 _]
    tunnel: w3 -> [w1067 w1076]
    tunnel: [w1066 w1076] -> w2
    frame False {
      n434 = call "CRYPrefix Curve Name.vi"("Type In"=w1068, "Curves In"=w1075, "Values In"=w1074, "Results In"=w1067, "Waves In"=w1073, "Repeat State Array In"=w1069) -> ("Curves Out"=w1072:T3, "Values Out"=w1071:T3, "Results Out"=w1066:T5, "Waves Out"=w1070:T7)  [unwired: 6 in]
    }
    frame True {
    }
  }
  n435 = call "CRYGet Type from Data.vi"("Waves"=w11, "Values"=w12, "Curves"=w13) -> ("Type"=→"Types Out":string[])  [unwired: 8 in]
  n436 = call "CRYInsert Socket.vi"("sOption2"=w27, "Step No."=w9, "sOption1"=w16, "Waves"=w11, "Results"=w2, "Values"=w12, "Curves"=w13) -> ("Inserted Names Out"=→"Inserted Names Out":string[])  [unwired: 4 in]
